vi "Data Logging Application.vi"() -> ()   [LabVIEW 2014]
doc: "This application allows the user to save any variables on the shared variable engine (NI SVE) in a TDMS file."
uses:
  <vilib>/Utility/miscctls.llb/LVRectTypeDef.ctl
  TypeDef/Q1 Message.ctl
  Support/Data Logger Global Variable.vi
  Supporting Folder/DV Prototype Global Variables.vi
  Support/Data logger Array Enqueue Function.vi
  Support/Global Variables/Recording Stop Watch.vi
  Support/Data logger Scalar Enqueue Function.vi
  <vilib>/Utility/NIReport.llb/NI_report.lvclass
  <userlib>/Notify Icon/Public/NotifyIcon.lvclass
panel:
  in  "DB Type":u16
  in  "delimiter":string=";"
  in  "Invisible Libraries":string[](array[string])
  in  "TDMS Properties":bool
  in  "Folder Setting":bool
  in  "Preference":bool
  in  "Description":string
  in  "Author":string
  in  "Title":string
  in  "Select All":bool
  in  "Auto Defrag":bool
  out "Date Time":string
  out "Application State":T1(ring)
  in  "Buffer size":u32=1000 min=1 step=1 format="%d data"
  in  "create database":bool
  out "Database Status":string
  in  "Deployed Libraries":i32[](listbox)
  in  "Server Name":string="localhost"
  in  "Add date/time to file name":bool
  in  "File Name":string="data log 1"
  out "Registered file name":string="data log 1" caption="Registered File Name"
  in  "database folder":path=path "C:/Ehsan Temp Folder/TFS/LV/Data Logging with LabVIEW/Database"
  in  "Folder to store TDMS file":path=path "C:/Ehsan Temp Folder/TFS/LV/Data Logging with LabVIEW/TDMS files"
  in  "View":bool
  in  "Initialize":bool
  in  "Stop Button":bool
  in  "Record Button":bool
  out "Recording Time":dbl format="%.1f sec"
  in  "Sampling Period":u32=100 min=1 step=1 format="%.0f msec"
  in  "Exit Button":bool
  in  "Variables":i32[](listbox)
  # "Data Logging Application"
  # "Status"
  # "Setting"
  # "Controls"
  # "Variables"
  # "Data Logging Application © 2015 Ehsan Peymani. All rights reserved."
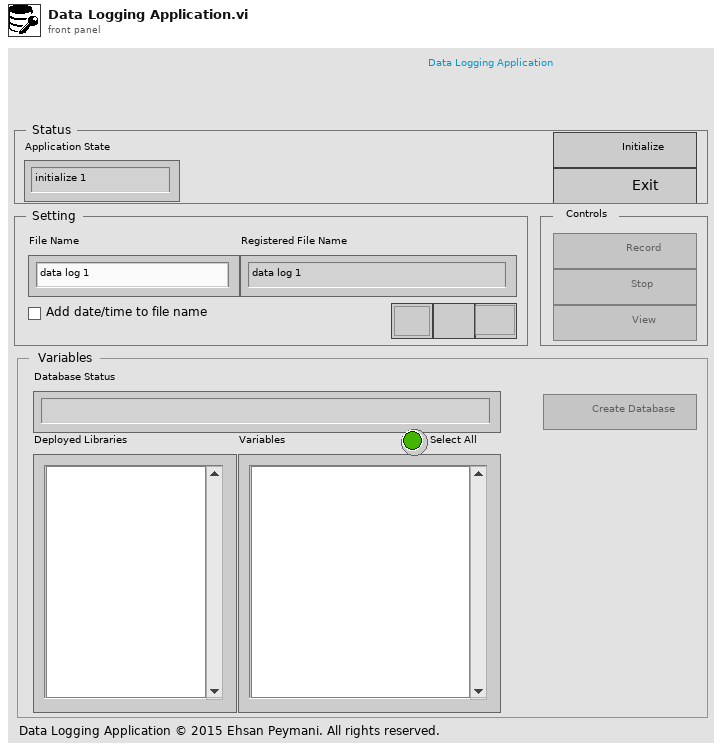
[diagram p1: front panel]
types:
  T1 = enum16{"initialize 1", "initialize 2", "initialize 3", "initialize 4", "initialize 5", "initialize 6", "initialize 7", "initialize 8", "initialize 9", "Idle", "Preparation 1", "Preparation 2", "Preparation 3", "Preparation 4", "Record", "Stop recording", "Exit", "Defrag", "View", "Create Database", "Update folder setting", "Update Preference", "Update TDMS properties", "CSV Delimiter", "DB Type", "Hidden Processes", "Replace Database", "Logged File Viewer", "Defrag Prompt File", "View Prompt File", "Save to config file", "Open from config file"}
  T2 = typedef "LVRectTypeDef.ctl" = cluster{"Left":i16, "Top":i16, "Right":i16, "Bottom":i16}
  T3 = enum16{"Config File", "Image File", "Word Template", "Release Note", "Help HTML", "Help Word", "Error List", "Excel Template", "CSV Template", "Tray Icon"}
  T4 = cluster{"Folder Path containing version information":path, "File name (including .ini)":path, "Section":string}
  T5 = typedef "LVPointTypeDef.ctl" = cluster{"Horizontal":i16, "Vertical":i16}
  T6 = cluster{"no. Displays":i32, "Display info - Menu":string[]}
  T7 = cluster{"path":path, "This VI":refnum<vi>, "Level of Application":u8}
  T8 = cluster{"Selected Variable Names":string[], "Selected Variable URL":string[], "Selected Variable Type":string[], "Container Variable Name":string[], "Container Variable URL":string[], "Selected Library URL":string[], "Library Name":string[], "Library URL":string[], "TDMS ref":refnum<k34>, "TDMS file path":path, "DB path array":path[], "DB availability for selected":bool[], "Selected Variables":i32[], "Bool Control Ref":refnum<vi>[], "Seetings ref":refnum<vi>[]}
  T9 = cluster{"String":refnum<vi>[], "Numeric":refnum<vi>[], "Path":refnum<vi>[], "Boolean":refnum<vi>[]}
  T10 = cluster{"Q2_scalar":refnum<queue>, "Q2_1Darray":refnum<queue>, "Q2_2Darray":refnum<queue>}
  T11 = enum32{"Invalid", "Standard", "Closed", "Hidden", "Minimized", "Maximized"}
  T12 = enum16{"Config File", "Image File", "Word Template", "Release Note", "Help HTML", "Help Word", "Error List", "Excel Template", "CSV Template"}
  T13 = typedef "Q1 Message.ctl" = cluster{"state":enum16{"initialize 1", "initialize 2", "initialize 3", "initialize 4", "initialize 5", "initialize 6", "initialize 7", "initialize 8", "initialize 9", "Idle", "Preparation 1", "Preparation 2", "Preparation 3", "Preparation 4", "Record", "Stop recording", "Exit", "Defrag", "View", "Create Database", "Update folder setting", "Update Preference", "Update TDMS properties", "CSV Delimiter", "DB Type", "Hidden Processes", "Replace Database", "Logged File Viewer", "Defrag Prompt File", "View Prompt File", "Save to config file", "Open from config file"}, "data":variant}
  T14 = enum16{"Standard Report", "HTML", "Word", "Excel"}
  T15 = enum16{"maximized", "minimized", "normal", "no change"}
  T16 = enum16{"Config File", "Image File", "Word Template", "Release Note", "Help HTML", "Help Word", "Error List", "Excel Template", "CSV Template", "Tray Icon", "Data Viewer"}
  T17 = typedef "sizeaction.ctl" = enum32{"Minimized", "Maximized", "Resized"}
  T18 = cluster{"Title":string, "Title":string, "Icon":i32, "Timeout (ms)":i32}
  T19 = typedef "Notify Icon.lvclass/Notify Event Type.ctl" = enum16{"<Invalid Event>", "Tray Icon Click", "Tray Icon DoubleClick", "BalloonTip Shown", "BalloonTip Clicked", "BalloonTip Closed", "Menu Item Clicked"}
  T20 = typedef "eventvkey.ctl" = enum16{"ASCII", "Enter", "Return", "Shift", "Ctrl", "Alt", "Cmd", "Opt", "Caps", "NumLock", "Clear", "Break", "Up", "Down", "Left", "Right", "Insert", "Delete", "Home", "End", "PageUp", "PageDown", "Escape", "Help", "Pause", "ScrollLock", "F1", "F2", "F3", "F4", "F5", "F6", "F7", "F8", "F9", "F10", "F11", "F12", "F13", "F14", "F15", "F16", "F17", "F18", "F19", "F20", "F21", "F22", "F23", "F24", "Play", "VolumeUp", "VolumeDown", "Mute", "Two Byte Char"}
  T21 = cluster{"Shift":bool, "Ctrl":bool, "Alt":bool, "Cmd":bool, "Opt":bool}
  T22 = enum8{"Enabled", "Disabled", "Disabled and Grayed Out"}
  T23 = enum16{"open", "open or create", "create or replace", "create", "open (read-only)"}
  T24 = cluster{"Library Name":string[], "library URL":string[]}
  T25 = cluster{"Variable Name":string[], "Variable URL":string[], "Variable Type":string[], "Variable Type Code":i32[]}
  T26 = cluster{"Sampling Period":u32, "TDMS ref":refnum<k34>, "Selected Variable URL":string[], "Selected Variable Type":string[], "Selected Variable Names":string[]}
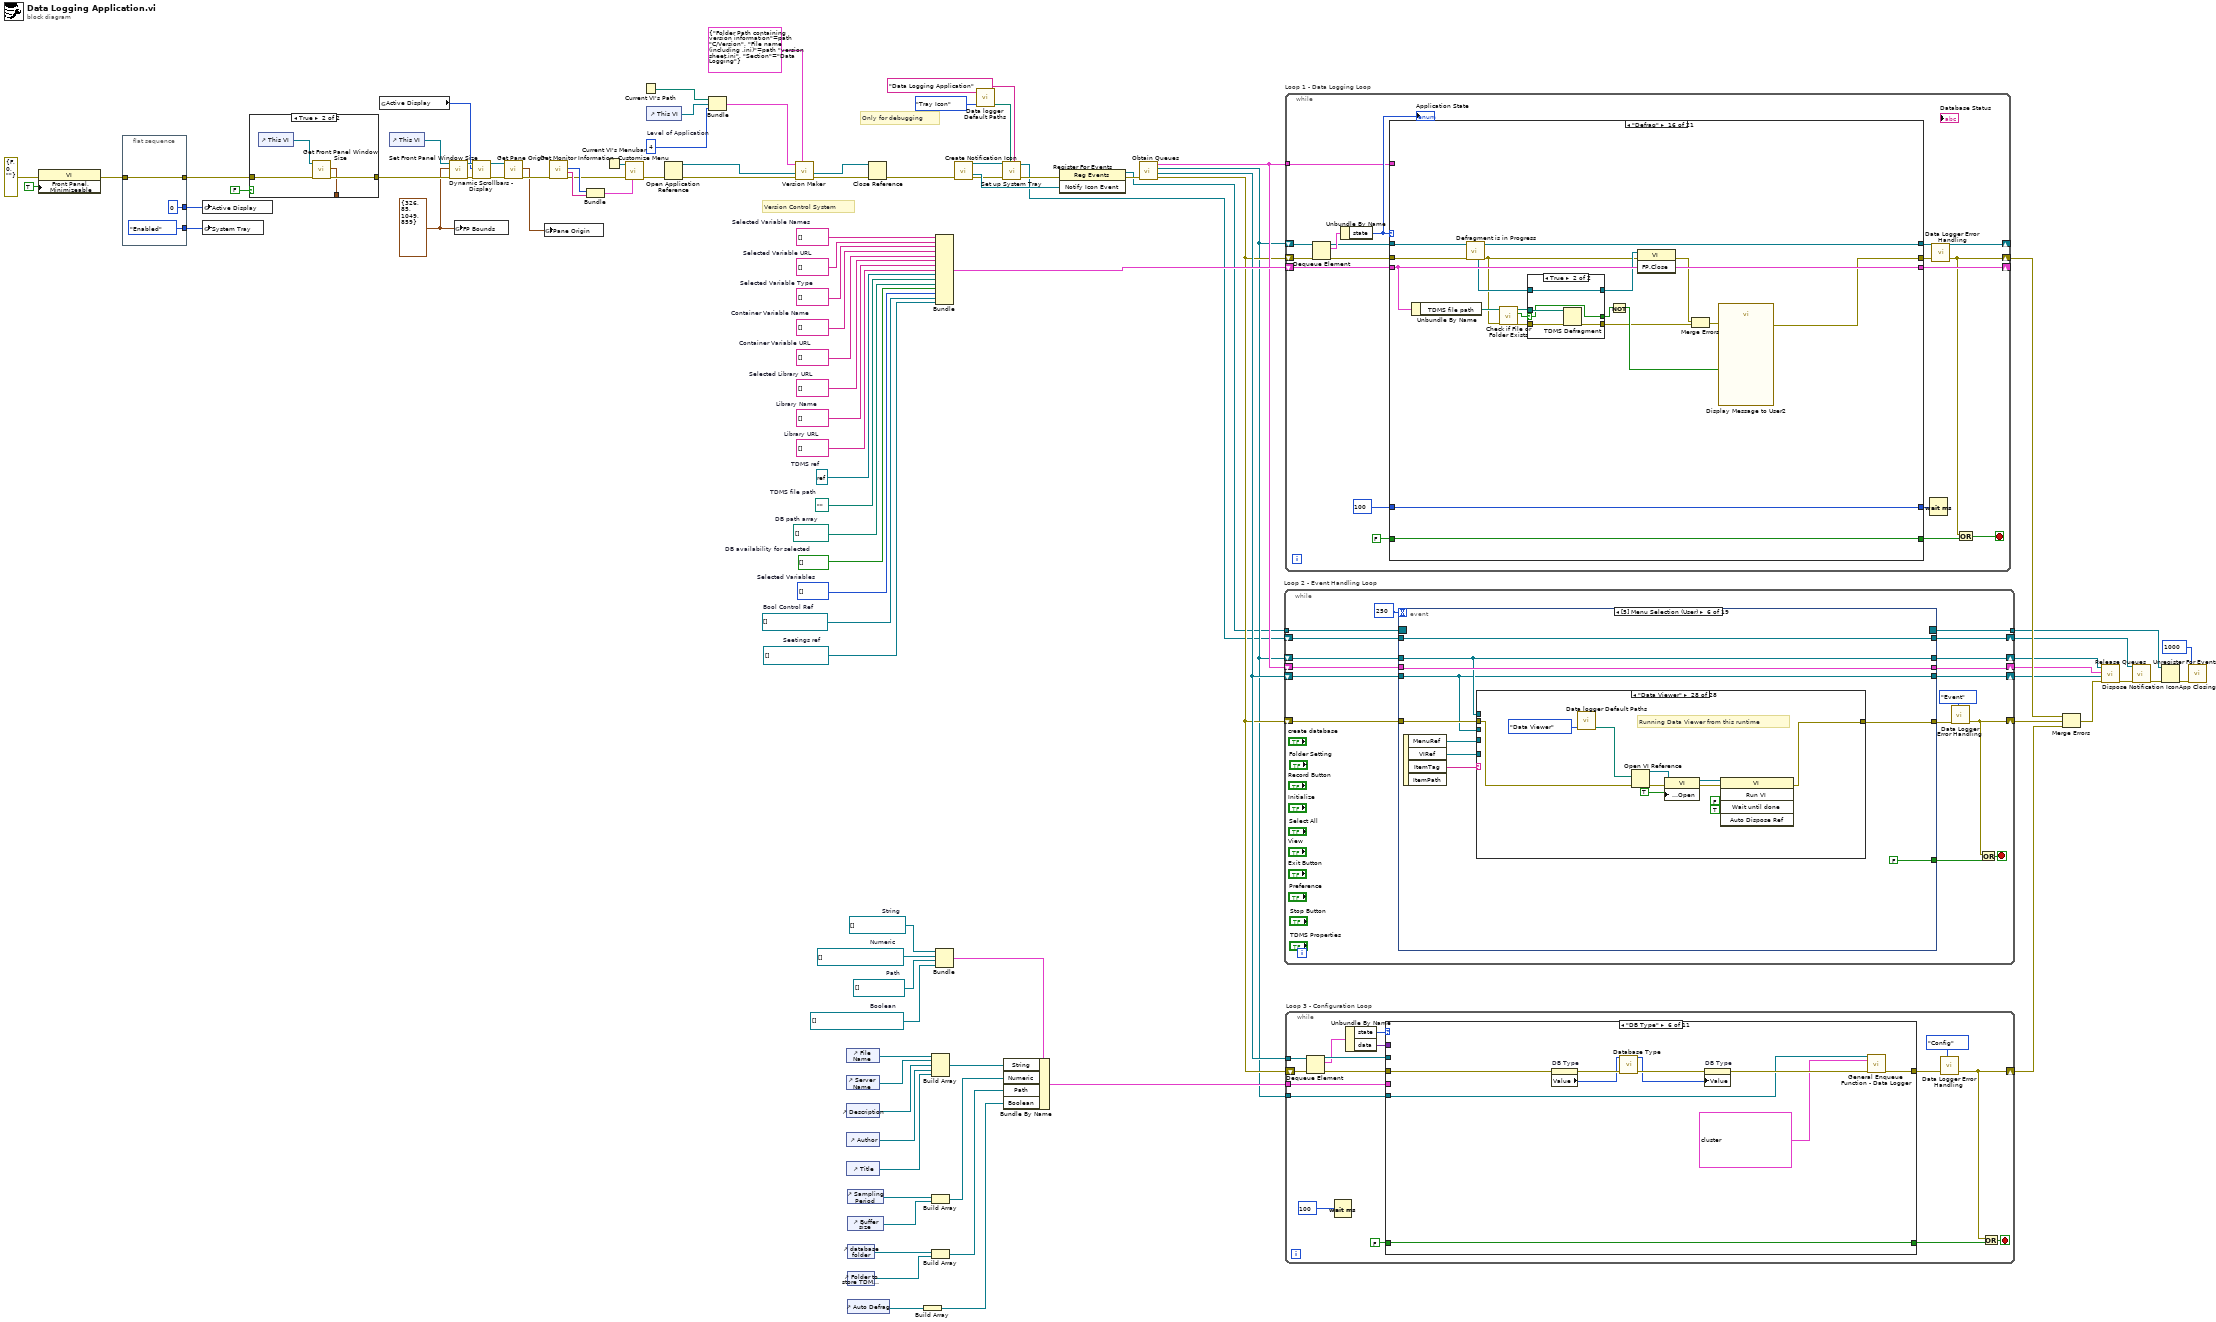
[diagram p0: block diagram]
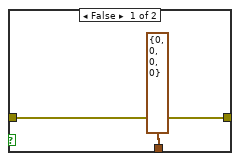
[diagram p2: hidden frame]
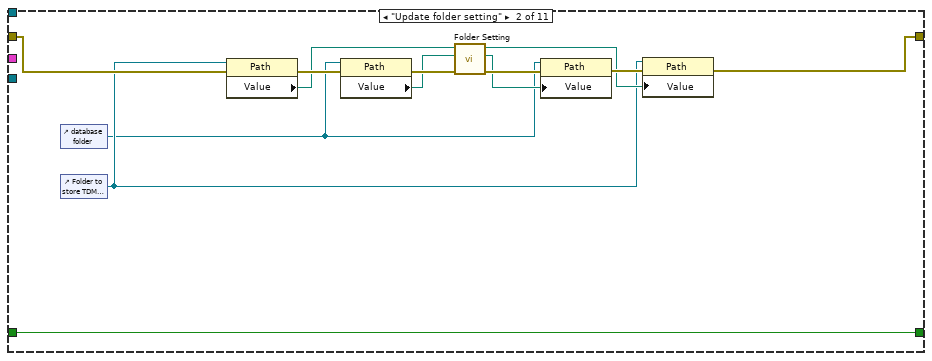
[diagram p4: hidden frame]
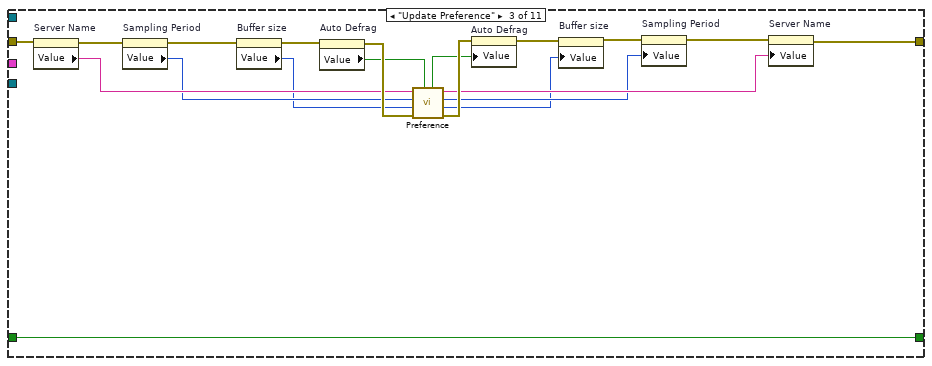
[diagram p5: hidden frame]
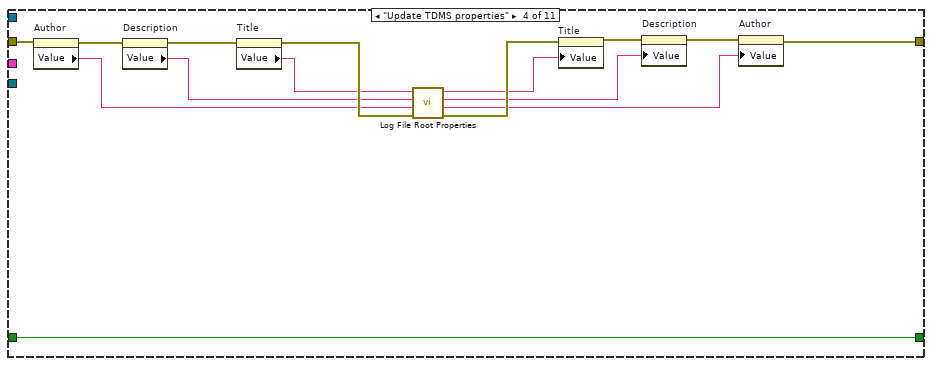
[diagram p6: hidden frame]
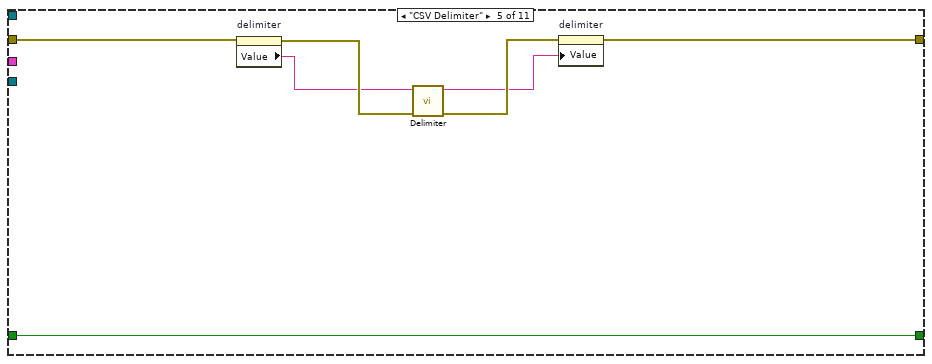
[diagram p7: hidden frame]
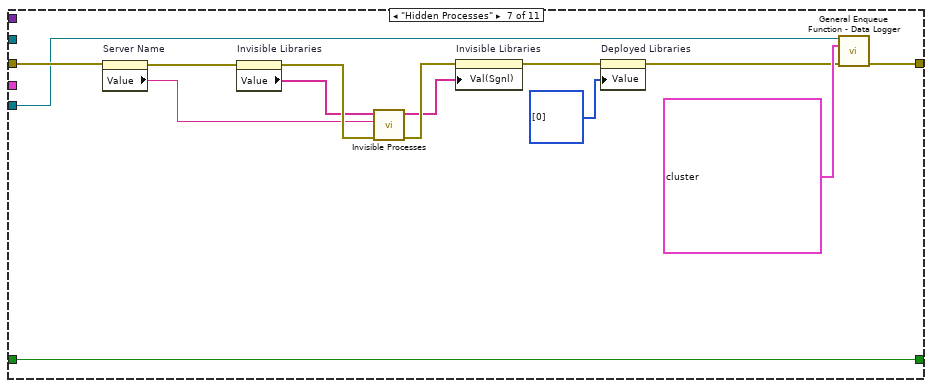
[diagram p8: hidden frame]
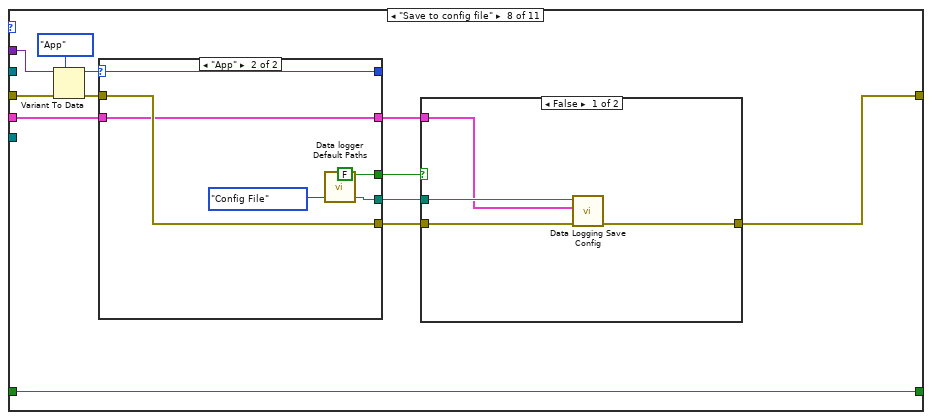
[diagram p9: hidden frame]
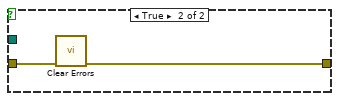
[diagram p10: hidden frame]
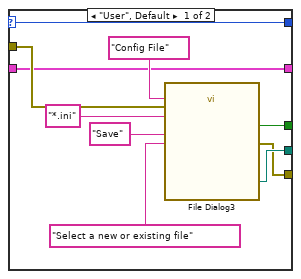
[diagram p11: hidden frame]
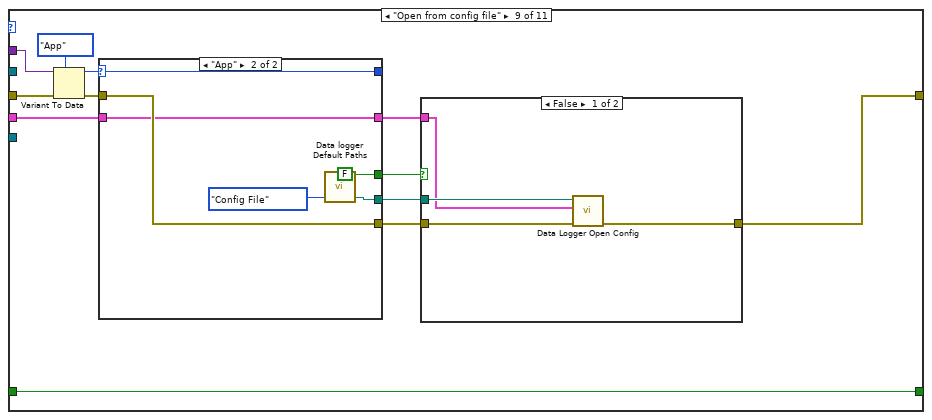
[diagram p12: hidden frame]
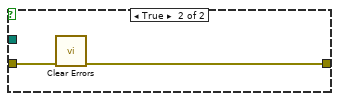
[diagram p13: hidden frame]
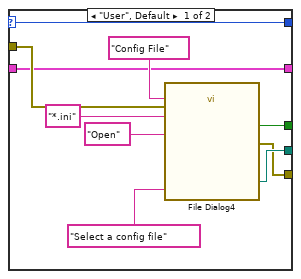
[diagram p14: hidden frame]
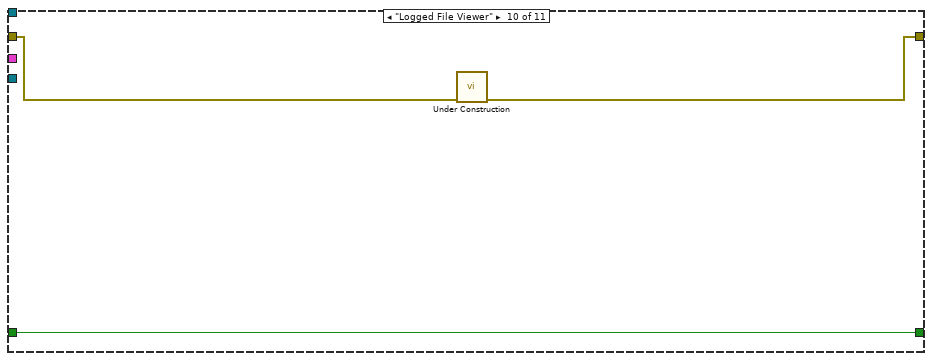
[diagram p15: hidden frame]
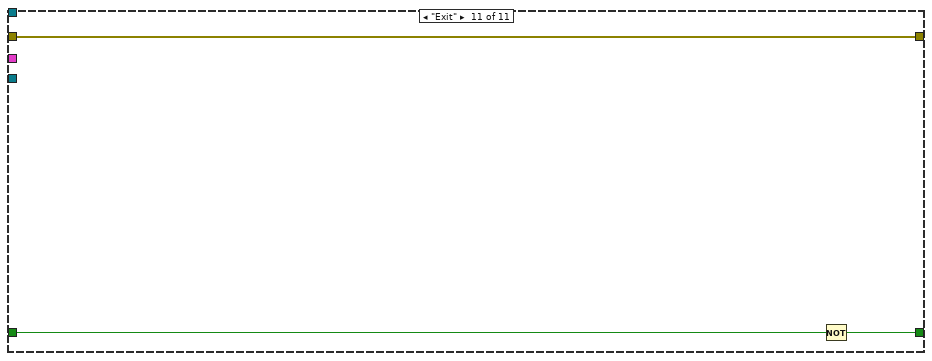
[diagram p16: hidden frame]
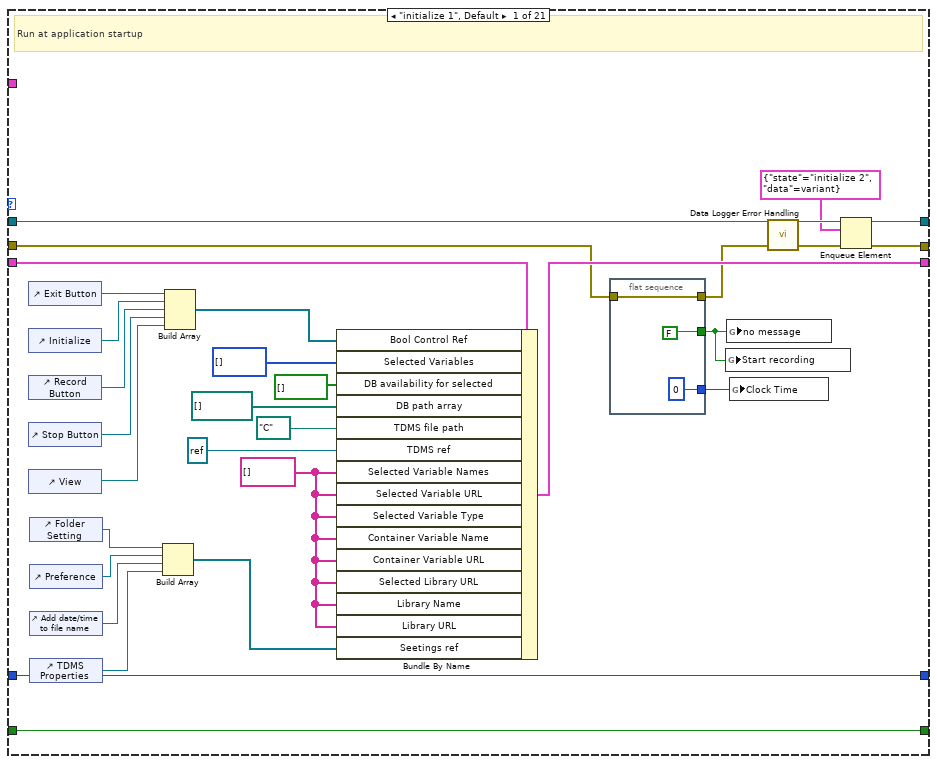
[diagram p17: hidden frame]
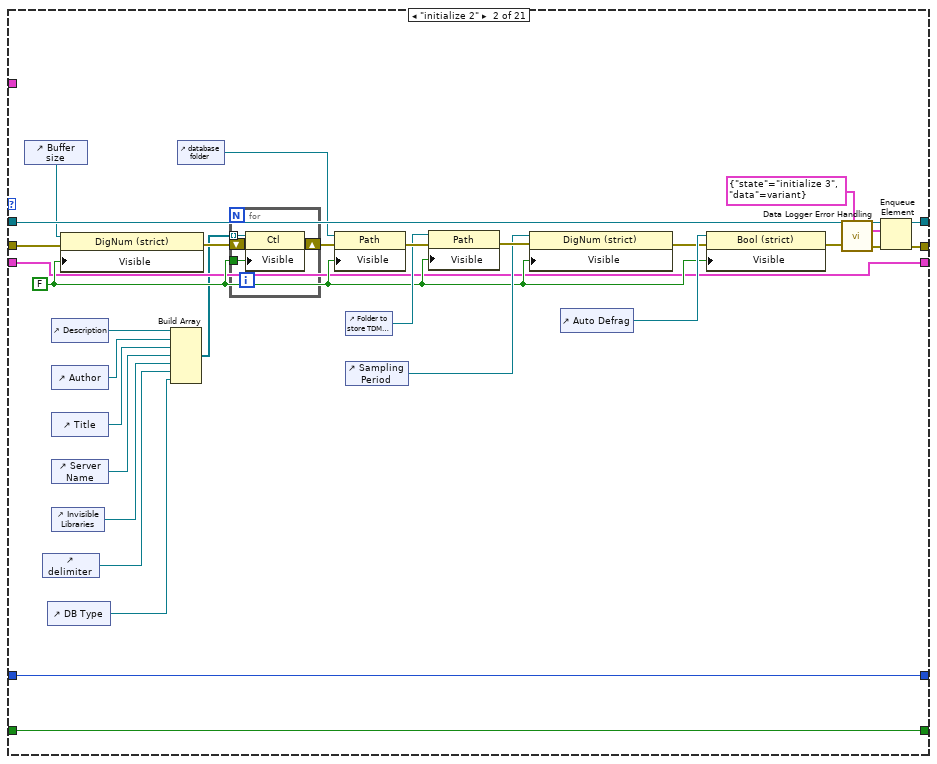
[diagram p18: hidden frame]
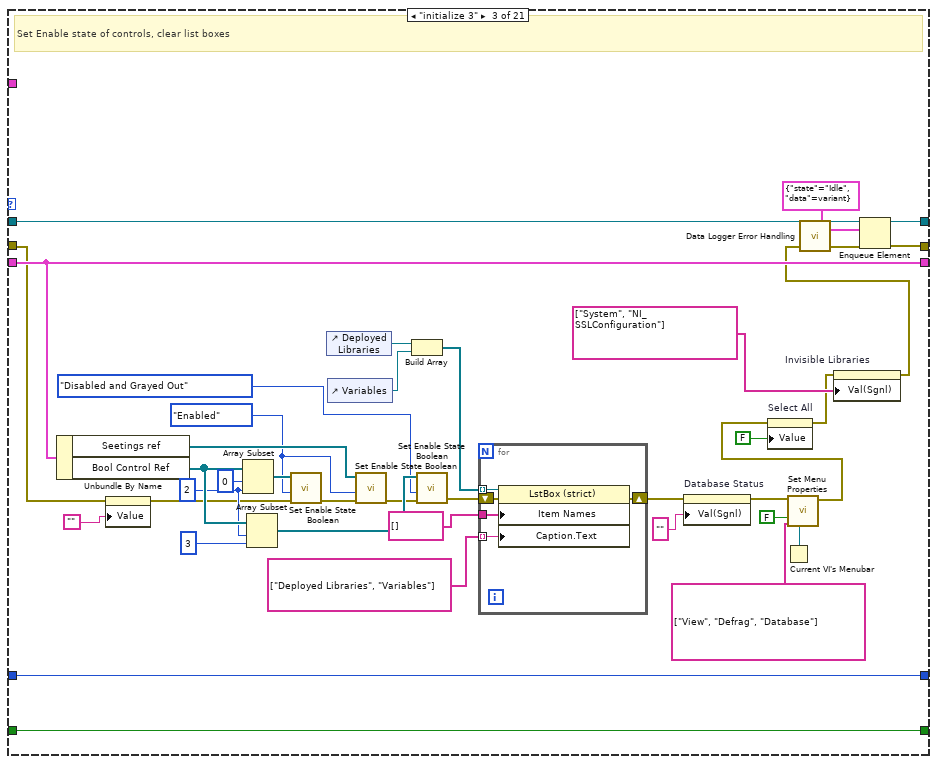
[diagram p19: hidden frame]
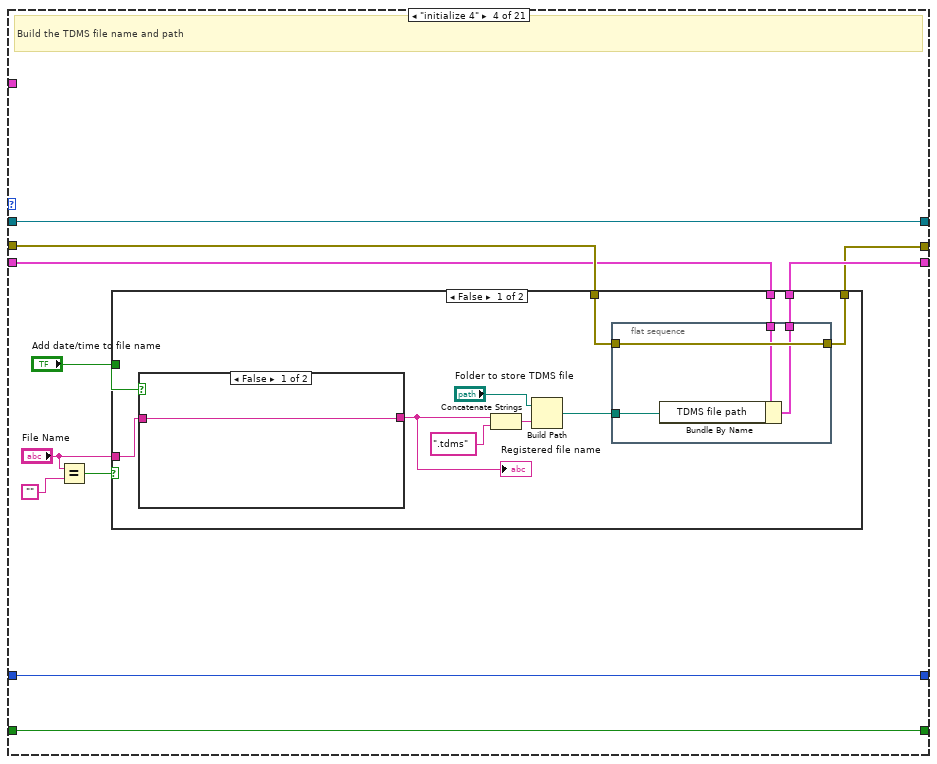
[diagram p20: hidden frame]
diagram:
  w5 = refnum<vi>[] []  # Seetings ref
  w7 = T2 {"Left"=326, "Top"=85, "Right"=1049, "Bottom"=859} ("Front Panel Window:Window Bounds")
  w45 = refnum<vi>[] []  # Boolean
  w48 = refnum<vi>[] []  # Numeric
  w51 = refnum<vi>[] []  # Path
  w54 = refnum<vi>[] []  # String
  w71 = string[] []  # Container Variable URL
  w80 = refnum<vi>[] []  # Bool Control Ref
  w75 = refnum<k34> refnum  # TDMS ref
  w79 = i32[] []  # Selected Variables
  w78 = bool[] []  # DB availability for selected
  w77 = path[] []  # DB path array
  w76 = path ""  # TDMS file path
  w74 = string[] []  # Library URL
  w73 = string[] []  # Library Name
  w72 = string[] []  # Selected Library URL
  w82 = string[] []  # Container Variable Name
  w83 = string[] []  # Selected Variable Type
  w84 = string[] []  # Selected Variable URL
  w85 = string[] []  # Selected Variable Names
  w88 = u8 4  # Level of Application
  # "Only for debugging"
  # "Version Control System"
  n1 = property class="VI"(error in=errorcluster {"status"=FALSE, "code"=0, "source"=""} ("error constant"), "Front Panel.Minimizeable"=TRUE ("Front Panel Window:Minimizable")) -> (error out=w4:errorcluster)  [unwired: 1 in, 1 out]
  n2 = flat-sequence {
    tunnel: [u16 0 ("Active Display")] -> w23
    tunnel: [enum16{"Enabled", "Disabled"}."Enabled" ("System Tray")] -> w22
    tunnel: [w97] -> w10
    tunnel: w4 -> [w97]
    frame #0 {
    }
  }
  n3 = global write "Data Logger Global Variable.vi" "Active Display"(w23) -> ()
  n4 = global write "Data Logger Global Variable.vi" "System Tray"(w22) -> ()
  n5 = case shown="True" FALSE {
    tunnel: w10 -> [w101 w104]
    tunnel: [w101 w103] -> w12
    tunnel: [T2 {"Left"=0, "Top"=0, "Right"=0, "Bottom"=0} ("Front Panel Window:Window Bounds") w102] -> _
    frame False {
    }
    frame True {
      n6 = control-ref of="This VI"() -> (w105:refnum<vi>)
      n7 = call "Get Front Panel Window Size.vi"("error in"=w104, "VI Ref"=w105) -> ("error out"=w103:errorcluster, "FP:Window Bounds"=w102:T2)  [unwired: 4 in, 4 out]
    }
  }
  n8 = global read "DV Prototype Global Variables.vi" "Active Display"() -> (w13:u16)
  n9 = control-ref of="This VI"() -> (w19:refnum<vi>)
  n10 = call "Set Front Panel Window Size.vi"("error in"=w12, "Front Panel Window:Window Bounds"=w7, "VI Ref"=w19) -> ("error out"=w21:errorcluster, "VI Ref"=w20:refnum<vi>)  [unwired: 7 in]
  n11 = global write "Data Logger Global Variable.vi" "FP Bounds"(w7) -> ()
  n12 = call "Dynamic Scrollbars - Display.vi"("error in"=w21, "Active Display in"=w13, "VI Ref"=w20) -> ("error out"=w18:errorcluster, "VI Ref"=w17:refnum<vi>)  [unwired: 6 in, 1 out]
  n13 = call "Get Pane Origin.vi"("error in"=w18, "VI Ref"=w17) -> ("error out"=w16:errorcluster, "Pane Origin"=w6:T5[])  [unwired: 7 in, 1 out]
  n14 = global write "Data Logger Global Variable.vi" "Pane Origin"(w6) -> ()
  n15 = call "Get Monitor Information.vi"("error in"=w16) -> ("error out"=w11:errorcluster, "Display info - Menu"=w14:string[], "no. Displays"=w15:i32)  [unwired: 6 in, 2 out]
  n16 = Bundle("no. Displays"=w15, "Display info - Menu"=w14) -> (w8:T6)  [unwired: 1 in]
  n17 = Current VI's Menubar() -> (w70:refnum<k9>)
  n18 = call "Customize Menu.vi"("Display information"=w8, "error in"=w11, "menu reference"=w70) -> ("error out"=w69:errorcluster)  [unwired: 8 in]
  n19 = Current VI's Path() -> (path=w86:path)
  n20 = control-ref of="This VI"() -> (w87:refnum<vi>)
  n21 = Open Application Reference(8:w69) -> (0:w94:errorcluster, 3:w91:refnum<vi>)  [unwired: 3 in]
  n22 = Bundle("path"=w86, "This VI"=w87, "Level of Application"=w88) -> (w89:T7)  [unwired: 1 in]
  n23 = call "Version Maker.vi"("Version Sheet Cluster"=T4 {"Folder Path containing version information"=path "C:/Version", "File name (including .ini)"=path "version sheet.ini", "Section"="Data Logging"}, "Error In"=w94, "Open Application Reference in"=w91, "VI Information"=w89) -> ("Error Out"=w93:errorcluster, "Open Application Reference out"=w90:refnum<vi>)  [unwired: 4 in, 2 out]
  n24 = control-ref of="File Name"() -> (w60:refnum<vi>)
  n25 = control-ref of="Server Name"() -> (w59:refnum<vi>)
  n26 = control-ref of="Description"() -> (w43:refnum<vi>)
  n27 = control-ref of="Author"() -> (w42:refnum<vi>)
  n28 = control-ref of="Title"() -> (w41:refnum<vi>)
  n29 = control-ref of="Sampling Period"() -> (w58:refnum<vi>)
  n30 = control-ref of="Buffer size"() -> (w57:refnum<vi>)
  n31 = control-ref of="database folder"() -> (w56:refnum<vi>)
  n32 = control-ref of="Folder to store TDMS file"() -> (w55:refnum<vi>)
  n33 = control-ref of="Auto Defrag"() -> (w46:refnum<vi>)
  n34 = Close Reference(reference=w90, error in (no error)=w93) -> (error out=w33:errorcluster)
  n35 = Build Array(w46) -> (w44:refnum<vi>[])
  n36 = Build Array(w60, w59, w43, w42, w41) -> (w53:refnum<vi>[])
  n37 = Build Array(w58, w57) -> (w47:refnum<vi>[])
  n38 = Build Array(w56, w55) -> (w50:refnum<vi>[])
  n39 = Bundle("Selected Variable Names"=w85, "Selected Variable URL"=w84, "Selected Variable Type"=w83, "Container Variable Name"=w82, "Container Variable URL"=w71, "Selected Library URL"=w72, "Library Name"=w73, "Library URL"=w74, "TDMS ref"=w75, "TDMS file path"=w76, "DB path array"=w77, "DB availability for selected"=w78, "Selected Variables"=w79, "Bool Control Ref"=w80, "Seetings ref"=w5) -> (w81:T8)  [unwired: 1 in]
  n40 = Bundle("String"=w54, "Numeric"=w48, "Path"=w51, "Boolean"=w45) -> (w52:T9)  [unwired: 1 in]
  n41 = call <userlib>:"Create Notification Icon.vi"("error in (no error)"=w33) -> ("NotifyIcon out"=w37:refnum<class "NotifyIcon.lvclass">, "Notify Icon Event"=w39:refnum<user-event>, "error out"=w38:errorcluster)  [unwired: 12 out]
  n42 = call "Data logger Default Paths.vi"("Path Type"=T3."Tray Icon") -> ("Path"=w31:path)  [unwired: 4 in]
  n43 = call "Set up System Tray.vi"("Icon Tip Strip Text"="Data Logging Application", "Image Path"=w31, "error in"=w38, "NotifyIcon in"=w37) -> ("error out"=w35:errorcluster, "NotifyIcon out"=w29:refnum<class "NotifyIcon.lvclass">)  [unwired: 6 in]
  n44 = Bundle By Name(cluster=w52, "String"=w53, "Numeric"=w47, "Path"=w50, "Boolean"=w44) -> (w49:T9)
  n45 = register-events(error in=w35, w39) -> (reference out=w30:refnum<event-registration>, error out=w34:errorcluster)  [unwired: 1 in]
  n46 = call "Obtain Queues.vi"("error in (no error)"=w34) -> ("error out"=w62:errorcluster, "Q3"=w63:refnum<queue>, "Q1"=w40:refnum<queue>, "Q2 Cluster"=w68:T10)  [unwired: 7 in]
  n47 = while "Loop 2 - Event Handling Loop" {
    shift-right: [w120] -> w66
    shift-left: w40 -> [w122]
    shift-right: [w111] -> w95
    shift-left: w62 -> [w121]
    shift-right: [w118] -> w65
    shift-left: w68 -> [w119]
    shift-right: [w113] -> w64
    shift-left: w63 -> [w114]
    tunnel: w30 -> [w109]
    shift-right: [w107] -> w25
    shift-left: w29 -> [w108]
    tunnel: [w106] -> w24
    stop <- w116 stop-if-true
    n48 = event shown="[5] Menu Selection (User)" {
      selector: w109 -> [_ _ _ _ _ _ _ _ _ _ _ _ _ _ _ _ _ _ _]
      dyn-events: [_ _ _ _ _ _ _ _ _ _ _ _ _ _ _ _ _ _ _] -> w106
      timeout: u32 250 ("milliseconds to wait") -> [_ _ _ _ _ _ _ _ _ _ _ _ _ _ _ _ _ _ _]
      tunnel: w122 -> [w134 w154 w163 w199 w242 w360 w563 w585 w595 w604 w613 w625 w637 w642 w654 w662 w670 w678 w701]
      tunnel: w121 -> [w128 w149 w160 w196 w244 w362 w576 w580 w590 w602 w612 w621 w636 w646 w650 w658 w666 w674 w690]
      tunnel: [_ _ _ _ w238 FALSE TRUE FALSE FALSE FALSE _ _ _ _ _ _ _ _ _] -> w117
      tunnel: [w134 w154 w163 w199 w242 w360 w562 w586 w595 w605 w616 w627 w638 w642 w654 w662 w670 w678 w701] -> w120
      tunnel: [w131 w149 w159 w195 w243 w361 w565 w584 w594 w607 w614 w628 w635 w643 w653 w661 w669 w673 w698] -> w112
      tunnel: w119 -> [w133 w153 w162 w198 w241 w364 w577 w587 w593 w608 w617 w631 w639 w647 w655 w663 w671 w677 w700]
      tunnel: [w133 w153 w162 w198 w241 w364 w577 w587 w593 w608 w617 w631 w639 w647 w655 w663 w671 w677 w700] -> w118
      tunnel: w114 -> [w124 w152 w161 w197 w240 w359 w575 w581 w591 w598 w611 w622 w633 w641 w652 w660 w668 w676 w699]
      tunnel: [w124 w152 w161 w197 w240 w359 w567 w581 w591 w598 w611 w622 w633 w641 w651 w659 w667 w676 w699] -> w113
      tunnel: w108 -> [w123 w151 w158 w194 w236 w357 w561 w579 w589 w597 w610 w618 w632 w640 w648 w656 w664 w672 w689]
      tunnel: [w123 w151 w157 w193 w236 w357 w561 w579 w589 w597 w610 w618 w632 w640 w648 w656 w664 w672 w689] -> w107
      event Timeout {
        n49 = event-data() -> ()  [unwired: 1 in, 2 out]
        n50 = flat-sequence {
          tunnel: [w136] -> w125
          tunnel: w128 -> [w135]
          tunnel: [w135] -> w126
          frame #0 {
            n51 = Get Date/Time In Seconds() -> (seconds since 1Jan1904=w137:timestamp)
            n52 = Format Date/Time String(time format string (%c)="%Y-%m-%d  %H:%M:%S", seconds (now)=w137) -> (date/time string=w136:string)  [unwired: 1 in]
          }
        }
        n53 = global read "Recording Stop Watch.vi" "Start recording"() -> (w132:bool)
        n54 = case shown="False" w132 {
          tunnel: [0.0 w144] -> w129
          tunnel: [FALSE TRUE] -> w130
          tunnel: [w139 w142] -> w127
          tunnel: w126 -> [w139 w142]
          frame False {
          }
          frame True {
            n55 = global read "Recording Stop Watch.vi" "Clock Time"() -> (w147:u32)
            n56 = Tick Count (ms)() -> (millisecond timer value=w148:u32)
            n57 = Subtract(x=w148, y=w147) -> (x-y=w146:u32)
            n58 = Divide(x=w146, y=u32 1000) -> (x/y=w144:dbl)
          }
        }
        "Recording Time" <- w129
        n59 = property on="Recording Time" class="DigNum (strict)"(error in=w127, "Visible"=w130) -> (error out=w131:errorcluster)  [unwired: 1 in, 1 out]
        "Date Time" <- w125
      }
      event Panel Close? {
        n60 = event-data() -> ()  [unwired: 1 in, 4 out]
        n61 = event-data("Discard?"=TRUE) -> ()  [unwired: 1 in, 1 out]
      }
      event Panel Resize {
        n62 = event-data() -> ("VIRef"=w156:refnum<vi>, "Act"=w155:T17)  [unwired: 1 in]
        n63 = case shown="\"Minimized\", Default" w155 {
          tunnel: w156 -> [w164 w183 w189]
          tunnel: w158 -> [w175 w180 w190]
          tunnel: w160 -> [w167 w182 w186]
          tunnel: [w176 w181 w191] -> w159
          tunnel: [w169 w180 w190] -> w157
          frame "Minimized", Default {
            w172 = 1 items=["None", "Info", "Warning", "Error"] ("Icon")
            n64 = property class="VI"(reference=w164, error in=w167, "Front Panel.Minimizeable"=FALSE ("Front Panel Window:Minimizable")) -> (error out=w166:errorcluster)  [unwired: 1 out]
            n65 = global read "Data Logger Global Variable.vi" "System Tray"() -> (w168:enum16{"Enabled", "Disabled"})
            n66 = Bundle("Title"="Data Logging Application", "Title"="Data Logging Application is running. Click on this icon to bring it up. ", "Icon"=w172, "Timeout (ms)"=2500) -> (w170:T18)  [unwired: 1 in]
            n67 = call "Front Panel to System Tray.vi"("Balloon Tip Information"=w170, "Mode"=w168, "error in"=w166, "VIRef"=w164, "NotifyIcon"=w175) -> ("error out"=w176:errorcluster, "NotifyIcon"=w169:refnum<class "NotifyIcon.lvclass">)  [unwired: 5 in]
          }
          frame "Maximized" {
            n68 = global read "Data Logger Global Variable.vi" "Pane Origin"() -> (w177:T5[])
            n69 = global read "Data Logger Global Variable.vi" "FP Bounds"() -> (w178:T2)
            n70 = global read "Data Logger Global Variable.vi" "Active Display"() -> (w179:u16)
            n71 = call "Reset Front Panel.vi"("Active Display"=w179, "error in"=w182, "Pane Origin"=w177, "Front Panel Bounds"=w178, "VI Ref"=w183) -> ("error out"=w181:errorcluster)  [unwired: 5 in, 1 out]
          }
          frame "Resized" {
            n72 = global read "Data Logger Global Variable.vi" "FP Bounds"() -> (w184:T2)
            n73 = call "Get Front Panel Window Size.vi"("error in"=w186, "VI Ref"=w189) -> ("error out"=w187:errorcluster, "FP:Window Bounds"=w185:T2, "VI Ref"=w188:refnum<vi>)  [unwired: 4 in, 3 out]
            n74 = call "Dynamic Scrollbars - Resize Front Panel.vi"("error in"=w187, "OrgBnds"=w184, "NewBnds"=w185, "VI Ref"=w188) -> ("error out"=w191:errorcluster)  [unwired: 6 in, 1 out]
          }
        }
      }
      event User Event {
        n75 = event-data() -> ("Type"=w192:T19)  [unwired: 1 in]
        n76 = case shown="\"Tray Icon Click\"" w192 {
          tunnel: w196 -> [w201 w205 w227 w229 w231 w233 w235]
          tunnel: [w201 w210 w227 w229 w231 w233 w235] -> w195
          tunnel: [w200 w209 w226 w228 w230 w232 w234] -> w193
          tunnel: w194 -> [w200 w208 w226 w228 w230 w232 w234]
          frame "<Invalid Event>", Default {
          }
          frame "Tray Icon Click" {
            n77 = control-ref of="This VI"() -> (w203:refnum<vi>)
            n78 = property class="VI"(reference=w203, error in=w205, "Front Panel.Minimizeable"=TRUE ("Front Panel Window:Minimizable")) -> (reference out=w202:refnum<vi>, error out=w206:errorcluster)
            n79 = property class="VI"(reference=w202, error in=w206) -> (reference out=w216:refnum<vi>, error out=w215:errorcluster, "FP.State"=w217:T11)
            n80 = case shown="\"Hidden\"" w217 {
              tunnel: w216 -> [w219 w225]
              tunnel: w215 -> [w218 w224]
              tunnel: T11."Standard" ("State") -> [_ w222]
              tunnel: [w218 w221] -> w213
              tunnel: [w219 w220] -> w212
              frame "Invalid", Default {
              }
              frame "Hidden" {
                n81 = invoke class="VI" method="FP.Open"(reference=w225, error in=w224, "Activate"=TRUE, "State"=w222) -> (reference out=w220:refnum<vi>, error out=w221:errorcluster)  [unwired: 1 in, 3 out]
              }
            }
            n82 = Close Reference(reference=w212, error in (no error)=w213) -> (error out=w211:errorcluster)
            n83 = call <userlib>:"Set Tray Icon Visibility.vi"("NotifyIcon in"=w208, "Show Tray Icon"=FALSE, "error in (no error)"=w211) -> ("NotifyIcon out"=w209:refnum<class "NotifyIcon.lvclass">, "error out"=w210:errorcluster)  [unwired: 11 out]
          }
          frame "Tray Icon DoubleClick" {
          }
          frame "BalloonTip Shown" {
          }
          frame "BalloonTip Clicked" {
          }
          frame "BalloonTip Closed" {
          }
          frame "Menu Item Clicked" {
          }
        }
      }
      event Key Down? {
        n84 = event-data() -> ("Char"=w247:i16, "VKey"=w248:T20, "PlatMods"=w249:T21)  [unwired: 1 in, 7 out]
        n85 = case shown="\"F1\"" w248 {
          tunnel: w247 -> [w344 _ _]
          tunnel: [w345 "" ("type") "" ("type")] -> w245
          tunnel: [w342 w347 w351] -> w250
          tunnel: w244 -> [w342 w347 w352]
          tunnel: T12."Help HTML" ("Path Type 2") -> [_ _ w349]
          frame "ASCII", Default {
            n86 = To Unsigned Byte Integer(number=w344) -> (unsigned 8bit integer=w343:u8)
            n87 = Type Cast(type="a", x=w343) -> (*(type *) &x=w345:string)
          }
          frame "Enter" {
          }
          frame "F1" {
            n88 = call "Data logger Default Paths.vi"("Path Type"=w349) -> ("Path"=w353:path)  [unwired: 4 in]
            n89 = Control Online Help(1:w352, 2:w353, 4:enum16{"Contents", "Key", "Close"}."Contents" ("Operation")) -> (0:w351:errorcluster)  [unwired: 1 in]
          }
        }
        n90 = Unbundle By Name(w249) -> ("Ctrl"=w246:bool)
        n91 = case shown="True" w246 {
          tunnel: w245 -> [_ w260]
          tunnel: w250 -> [w252 w259]
          tunnel: [w252 w258] -> w243
          tunnel: w242 -> [_ w257]
          tunnel: w241 -> [_ w256]
          tunnel: w240 -> [_ w255]
          tunnel: FALSE -> [w251 w254]
          tunnel: [w251 w253] -> w238
          frame False {
          }
          frame True {
            n92 = case shown="\"E\", \"Q\", \"e\", \"q\"" w260 {
              tunnel: w259 -> [w262 w267 w273 w287 w298 w309 w322]
              tunnel: [w262 w263 w276 w290 w301 w312 w324] -> w258
              tunnel: w257 -> [_ _ w275 w289 w300 _ w323]
              tunnel: w256 -> [_ _ _ _ _ w311 _]
              tunnel: w255 -> [_ _ _ _ _ _ w325]
              tunnel: w254 -> [w261 w268 w274 w288 w299 w310 w319]
              tunnel: [w261 w268 w274 w288 w299 w310 w318] -> w253
              frame "False", Default {
              }
              frame "A", "a" {
                n93 = property on="Select All" class="Bool (strict)"(error in=w267) -> (error out=w264:errorcluster, "Value"=w266:bool)  [unwired: 1 in, 1 out]
                n94 = Not(x=w266) -> (.not. x?=w265:bool)
                n95 = property on="Select All" class="Bool (strict)"(error in=w264, "Val(Sgnl)"=w265) -> (error out=w263:errorcluster)  [unwired: 1 in, 1 out]
              }
              frame "I", "i" {
                n96 = control-ref of="Initialize"() -> (w272:refnum<vi>)
                n97 = property class="Bool"(reference=w272, error in=w273) -> (reference out=w269:refnum<vi>, error out=w270:errorcluster, "DisabledEnum"=w271:T22)
                n98 = case shown="\"Disabled\", Default" w271 {
                  tunnel: [w277 w283] -> w276
                  tunnel: w275 -> [_ w280]
                  tunnel: w270 -> [w277 w278]
                  tunnel: w269 -> [_ w279]
                  frame "Disabled", Default {
                  }
                  frame "Enabled" {
                    n99 = property class="Bool"(reference=w279, error in=w278, "Blinking"=FALSE) -> (error out=w282:errorcluster)  [unwired: 1 out]
                    n100 = call-poly "General Enqueue Function - Data Logger.vi"("QRef in"=w280, "Array of Messages"=T13[] [{"state"=enum."initialize 3", "data"=variant}, {"state"=enum."initialize 4", "data"=variant}, {"state"=enum."initialize 5", "data"=variant}, {"state"=enum."initialize 6", "data"=variant}, {"state"=enum."Idle", "data"=variant}], "Error in"=w282) -> ("Error out"=w283:errorcluster)  [unwired: 11 in, 1 out]
                  }
                }
              }
              frame "R", "r" {
                n101 = property on="Record Button" class="Bool"(error in=w287) -> (error out=w286:errorcluster, "DisabledEnum"=w285:T22)  [unwired: 1 in, 1 out]
                n102 = case shown="\"Enabled\"" w285 {
                  tunnel: [w291 w295] -> w290
                  tunnel: w289 -> [_ w294]
                  tunnel: w286 -> [w291 w292]
                  frame "Disabled", Default {
                  }
                  frame "Enabled" {
                    n103 = call-poly "General Enqueue Function - Data Logger.vi"("QRef in"=w294, "Array of Messages"=T13[] [{"state"=enum."Preparation 1", "data"=variant}, {"state"=enum."Preparation 2", "data"=variant}, {"state"=enum."Preparation 3", "data"=variant}, {"state"=enum."Preparation 4", "data"=variant}, {"state"=enum."Record", "data"=variant}], "Error in"=w292) -> ("Error out"=w295:errorcluster)  [unwired: 11 in, 1 out]
                  }
                }
              }
              frame "V", "v" {
                n104 = property on="View" class="Bool"(error in=w298) -> (error out=w297:errorcluster, "DisabledEnum"=w296:T22)  [unwired: 1 in, 1 out]
                n105 = case shown="\"Enabled\"" w296 {
                  tunnel: [w305 w306] -> w301
                  tunnel: w300 -> [w304 _]
                  tunnel: w297 -> [w303 w306]
                  frame "Enabled" {
                    n106 = call-poly "General Enqueue Function - Data Logger.vi"("QRef in"=w304, "Q1 Message"=T13 {"state"=enum."View", "data"=variant}, "Error in"=w303) -> ("Error out"=w305:errorcluster)  [unwired: 11 in, 1 out]
                  }
                  frame "Disabled", Default {
                  }
                }
              }
              frame "S", "s" {
                n107 = property on="Stop Button" class="Bool"(error in=w309) -> (error out=w307:errorcluster, "DisabledEnum"=w308:T22)  [unwired: 1 in, 1 out]
                n108 = case shown="\"Enabled\"" w308 {
                  tunnel: [w316 w317] -> w312
                  tunnel: w307 -> [w315 w317]
                  tunnel: w311 -> [w314 _]
                  frame "Enabled" {
                    n109 = call "Enqueue Q2.vi"("Q1 Message"=T13 {"state"=enum."Stop recording", "data"=variant}, "error in (no error)"=w315, "Queue Ref"=w314) -> ("error out"=w316:errorcluster)  [unwired: 5 in, 3 out]
                  }
                  frame "Disabled", Default {
                  }
                }
              }
              frame "E", "Q", "e", "q" {
                n110 = property on="Exit Button" class="Bool"(error in=w322) -> (error out=w321:errorcluster, "DisabledEnum"=w320:T22)  [unwired: 1 in, 1 out]
                n111 = case shown="\"Enabled\"" w320 {
                  tunnel: w321 -> [w334 w341]
                  tunnel: w325 -> [w332 _]
                  tunnel: [w331 w341] -> w324
                  tunnel: w323 -> [w328 _]
                  tunnel: w319 -> [w327 w340]
                  tunnel: [w326 w340] -> w318
                  frame "Enabled" {
                    n112 = To Variant(anything=enum16{"App", "User"}."App") -> (Variant=w337:variant)
                    n113 = Bundle By Name(cluster=T13 {"state"=enum."Save to config file", "data"=variant} ("Q1 Message"), "data"=w337) -> (w338:T13)
                    n114 = Build Array(w338, T13 {"state"=enum."Exit", "data"=variant} ("Q1 Message")) -> (w333:T13[])
                    n115 = call-poly "General Enqueue Function - Data Logger.vi"("QRef in"=w332, "Array of Messages"=w333, "Error in"=w334) -> ("Error out"=w330:errorcluster)  [unwired: 11 in, 1 out]
                    n116 = Not(x=w327) -> (.not. x?=w326:bool)
                    n117 = call-poly "General Enqueue Function - Data Logger.vi"("QRef in"=w328, "Array of Messages"=T13[] [{"state"=enum."Exit", "data"=variant}], "Error in"=w330) -> ("Error out"=w331:errorcluster)  [unwired: 11 in, 1 out]
                  }
                  frame "Disabled", Default {
                  }
                }
              }
            }
          }
        }
        n118 = event-data() -> ()  [unwired: 2 in, 1 out]
      }
      event Menu Selection (User) {
        n119 = event-data() -> ("MenuRef"=w356:refnum<k9>, "VIRef"=w355:refnum<vi>, "ItemTag"=w363:string)  [unwired: 1 in, 1 out]
        n120 = case shown="\"Data Viewer\"" w363 {
          selector: w363 -> [_ _ _ _ _ _ _ _ _ _ _ _ _ _ _ _ _ _ _ _ _ _ w486 w494 w508 w522 w536 _]
          tunnel: w362 -> [w365 w369 w371 w373 w378 w384 w389 w394 w399 w404 w409 w414 w419 w424 w429 w434 w444 w454 w459 w462 w474 w480 w488 w496 w510 w524 w538 w553]
          tunnel: [w365 w368 w370 w375 w380 w385 w390 w395 w400 w405 w410 w415 w420 w425 w430 w435 w445 w455 w458 w463 w471 w481 w487 w495 w509 w523 w537 w552] -> w361
          tunnel: w360 -> [_ _ _ w374 w379 _ _ _ _ _ _ w411 _ w421 w426 w431 _ _ _ _ _ _ _ _ _ _ _ _]
          tunnel: w359 -> [_ _ _ _ _ w381 w386 w391 w396 w401 w406 _ w416 _ _ _ w442 w452 _ _ _ _ _ _ _ _ _ _]
          tunnel: w356 -> [_ _ _ _ _ _ _ _ _ _ _ _ _ _ _ _ _ _ _ _ _ _ w483 w497 w511 w525 w539 _]
          tunnel: w355 -> [_ _ _ _ _ _ _ _ _ _ _ _ _ _ _ _ _ _ _ _ _ _ _ w498 w512 w526 w540 _]
          frame "False", Default {
          }
          frame "Release Note" {
            n121 = call "Data logger Default Paths.vi"("Path Type"=T12."Release Note") -> ("Path"=w367:path)  [unwired: 4 in]
            n122 = call "open in notepad.vi"("error in (no error)"=w369, "Path"=w367) -> ("error out"=w368:errorcluster)  [unwired: 9 in]
          }
          frame "About Data Logging Application" {
            n123 = call "About Data Logger.vi"("Error In"=w371) -> ("Error Out"=w370:errorcluster)  [unwired: 10 in]
          }
          frame "View Current TDMS file" {
            n124 = call-poly "General Enqueue Function - Data Logger.vi"("QRef in"=w374, "Array of Messages"=T13[] [{"state"=enum."View", "data"=variant}, {"state"=enum."Idle", "data"=variant}], "Error in"=w373) -> ("Error out"=w375:errorcluster)  [unwired: 11 in, 1 out]
          }
          frame "Defrag Current TDMS file" {
            n125 = call-poly "General Enqueue Function - Data Logger.vi"("QRef in"=w379, "Array of Messages"=T13[] [{"state"=enum."Defrag", "data"=variant}, {"state"=enum."Idle", "data"=variant}], "Error in"=w378, "Mode"=enum16{"Back", "Front", "Replace"}."Replace") -> ("Error out"=w380:errorcluster)  [unwired: 10 in, 1 out]
          }
          frame "Folder Setting" {
            n126 = call-poly "General Enqueue Function - Data Logger.vi"("QRef in"=w381, "Array of Messages"=T13[] [{"state"=enum."Update folder setting", "data"=variant}, {"state"=enum."Idle", "data"=variant}], "Error in"=w384, "Mode"=enum16{"Back", "Front", "Replace"}."Replace") -> ("Error out"=w385:errorcluster)  [unwired: 10 in, 1 out]
          }
          frame "Preference" {
            n127 = call-poly "General Enqueue Function - Data Logger.vi"("QRef in"=w386, "Array of Messages"=T13[] [{"state"=enum."Update Preference", "data"=variant}, {"state"=enum."Idle", "data"=variant}], "Error in"=w389, "Mode"=enum16{"Back", "Front", "Replace"}."Replace") -> ("Error out"=w390:errorcluster)  [unwired: 10 in, 1 out]
          }
          frame "Log File Properties" {
            n128 = call-poly "General Enqueue Function - Data Logger.vi"("QRef in"=w391, "Array of Messages"=T13[] [{"state"=enum."Update TDMS properties", "data"=variant}, {"state"=enum."Idle", "data"=variant}], "Error in"=w394, "Mode"=enum16{"Back", "Front", "Replace"}."Replace") -> ("Error out"=w395:errorcluster)  [unwired: 10 in, 1 out]
          }
          frame "CSV Delimiter" {
            n129 = call-poly "General Enqueue Function - Data Logger.vi"("QRef in"=w396, "Array of Messages"=T13[] [{"state"=enum."CSV Delimiter", "data"=variant}, {"state"=enum."Idle", "data"=variant}], "Error in"=w399, "Mode"=enum16{"Back", "Front", "Replace"}."Replace") -> ("Error out"=w400:errorcluster)  [unwired: 10 in, 1 out]
          }
          frame "Database Type" {
            n130 = call-poly "General Enqueue Function - Data Logger.vi"("QRef in"=w401, "Array of Messages"=T13[] [{"state"=enum."DB Type", "data"=variant}, {"state"=enum."Idle", "data"=variant}], "Error in"=w404, "Mode"=enum16{"Back", "Front", "Replace"}."Replace") -> ("Error out"=w405:errorcluster)  [unwired: 10 in, 1 out]
          }
          frame "Hidden Processes" {
            n131 = call-poly "General Enqueue Function - Data Logger.vi"("QRef in"=w406, "Array of Messages"=T13[] [{"state"=enum."Hidden Processes", "data"=variant}, {"state"=enum."Idle", "data"=variant}], "Error in"=w409, "Mode"=enum16{"Back", "Front", "Replace"}."Replace") -> ("Error out"=w410:errorcluster)  [unwired: 10 in, 1 out]
          }
          frame "Replace the existing database" {
            n132 = call-poly "General Enqueue Function - Data Logger.vi"("QRef in"=w411, "Array of Messages"=T13[] [{"state"=enum."Replace Database", "data"=variant}, {"state"=enum."Idle", "data"=variant}], "Error in"=w414, "Mode"=enum16{"Back", "Front", "Replace"}."Replace") -> ("Error out"=w415:errorcluster)  [unwired: 10 in, 1 out]
          }
          frame "[Logged] Data Viewer" {
            n133 = call-poly "General Enqueue Function - Data Logger.vi"("QRef in"=w416, "Array of Messages"=T13[] [{"state"=enum."Logged File Viewer", "data"=variant}, {"state"=enum."Idle", "data"=variant}], "Error in"=w419, "Mode"=enum16{"Back", "Front", "Replace"}."Replace") -> ("Error out"=w420:errorcluster)  [unwired: 10 in, 1 out]
          }
          frame "Defrag Prompt TDMS file" {
            n134 = call-poly "General Enqueue Function - Data Logger.vi"("QRef in"=w421, "Array of Messages"=T13[] [{"state"=enum."Defrag Prompt File", "data"=variant}, {"state"=enum."Idle", "data"=variant}], "Error in"=w424, "Mode"=enum16{"Back", "Front", "Replace"}."Replace") -> ("Error out"=w425:errorcluster)  [unwired: 10 in, 1 out]
          }
          frame "View Prompt TDMS file" {
            n135 = call-poly "General Enqueue Function - Data Logger.vi"("QRef in"=w426, "Array of Messages"=T13[] [{"state"=enum."View Prompt File", "data"=variant}, {"state"=enum."Idle", "data"=variant}], "Error in"=w429, "Mode"=enum16{"Back", "Front", "Replace"}."Replace") -> ("Error out"=w430:errorcluster)  [unwired: 10 in, 1 out]
          }
          frame "Create missing database" {
            n136 = call-poly "General Enqueue Function - Data Logger.vi"("QRef in"=w431, "Array of Messages"=T13[] [{"state"=enum."Create Database", "data"=variant}, {"state"=enum."Idle", "data"=variant}], "Error in"=w434, "Mode"=enum16{"Back", "Front", "Replace"}."Replace") -> ("Error out"=w435:errorcluster)  [unwired: 10 in, 1 out]
          }
          frame "Save Configuration" {
            n137 = To Variant(anything=enum16{"App", "User"}."User") -> (Variant=w440:variant)
            n138 = Bundle By Name(cluster=T13 {"state"=enum."Save to config file", "data"=variant} ("Q1 Message"), "data"=w440) -> (w436:T13)
            n139 = Build Array(w436, T13 {"state"=enum."Idle", "data"=variant} ("Q1 Message")) -> (w438:T13[])
            n140 = call-poly "General Enqueue Function - Data Logger.vi"("QRef in"=w442, "Array of Messages"=w438, "Error in"=w444, "Mode"=enum16{"Back", "Front", "Replace"}."Replace") -> ("Error out"=w445:errorcluster)  [unwired: 10 in, 1 out]
          }
          frame "Load Configuration" {
            n141 = To Variant(anything=enum16{"App", "User"}."User") -> (Variant=w450:variant)
            n142 = Bundle By Name(cluster=T13 {"state"=enum."Open from config file", "data"=variant} ("Q1 Message"), "data"=w450) -> (w446:T13)
            n143 = Build Array(w446, T13 {"state"=enum."Idle", "data"=variant} ("Q1 Message")) -> (w448:T13[])
            n144 = call-poly "General Enqueue Function - Data Logger.vi"("QRef in"=w452, "Array of Messages"=w448, "Error in"=w454, "Mode"=enum16{"Back", "Front", "Replace"}."Replace") -> ("Error out"=w455:errorcluster)  [unwired: 10 in, 1 out]
          }
          frame "HTML" {
            n145 = call "Data logger Default Paths.vi"("Path Type"=T12."Help HTML") -> ("Path"=w457:path)  [unwired: 4 in]
            n146 = Control Online Help(1:w459, 2:w457, 4:enum16{"Contents", "Key", "Close"}."Contents" ("Operation")) -> (0:w458:errorcluster)  [unwired: 1 in]
          }
          frame "Excel Template" {
            n147 = call "Data logger Default Paths.vi"("Path Type"=T12."Excel Template") -> ("Path"=w467:path)  [unwired: 4 in]
            n148 = call <vilib>:"New Report.vi"("window state (normal)"=T15."maximized", "report type"=T14."Excel", "template (empty)"=w467, "error in (no error)"=w462) -> ("report out"=w466:refnum<class "NI_report.lvclass">, "error out"=w465:errorcluster)  [unwired: 10 in]
            n149 = call-dynamic "Dispose Report.vi"("report in"=w466, "error in (no error)"=w465, "close report? (T)"=FALSE) -> ("error out"=w463:errorcluster)  [unwired: 12 in]
          }
          frame "MS Word doc" {
            n150 = call "Data logger Default Paths.vi"("Path Type"=T12."Help Word") -> ("Path"=w472:path)  [unwired: 4 in]
            n151 = call <vilib>:"New Report.vi"("window state (normal)"=T15."maximized", "report type"=T14."Word", "template (empty)"=w472, "error in (no error)"=w474) -> ("report out"=w476:refnum<class "NI_report.lvclass">, "error out"=w475:errorcluster)  [unwired: 10 in]
            n152 = call-dynamic "Dispose Report.vi"("report in"=w476, "error in (no error)"=w475, "close report? (T)"=FALSE) -> ("error out"=w471:errorcluster)  [unwired: 12 in]
          }
          frame "CSV Template" {
            n153 = call "Data logger Default Paths.vi"("Path Type"=T12."CSV Template") -> ("Path"=w482:path)  [unwired: 4 in]
            n154 = call "open in notepad.vi"("error in (no error)"=w480, "Path"=w482) -> ("error out"=w481:errorcluster)  [unwired: 9 in]
          }
          frame "Tray" {
            n155 = global read "Data Logger Global Variable.vi" "System Tray"() -> (w485:enum16{"Enabled", "Disabled"})
            n156 = case shown="\"Disabled\"" w485 {
              tunnel: [enum16{"Enabled", "Disabled"}."Disabled" ("System Tray") enum16{"Enabled", "Disabled"}."Enabled" ("System Tray")] -> w484
              tunnel: ["System Tray: Disabled" "System Tray: Enabled"] -> w489
              frame "Enabled", Default {
              }
              frame "Disabled" {
              }
            }
            n157 = global write "Data Logger Global Variable.vi" "System Tray"(w484) -> ()
            n158 = Set Menu Item Info(7:w486, 8:w488, 10:w489, 11:w483) -> (0:w487:errorcluster)  [unwired: 3 in, 1 out]
          }
          frame "Display 0" {
            n159 = global read "Data Logger Global Variable.vi" "Active Display"() -> (w502:u16)
            n160 = flat-sequence {
              tunnel: w502 -> [w506]
              tunnel: [u16 0 ("Active Display")] -> w501
              tunnel: [w506] -> w503
              frame #0 {
              }
            }
            n161 = global write "Data Logger Global Variable.vi" "Active Display"(w501) -> ()
            n162 = global read "Data Logger Global Variable.vi" "FP Bounds"() -> (w500:T2)
            n163 = global read "Data Logger Global Variable.vi" "Pane Origin"() -> (w499:T5[])
            n164 = call "Display on Menu - Action.vi"("Item Tag"=w494, "Previous Active Display"=w503, "Active Display"=w501, "error in"=w496, "MenuRef"=w497, "FP Bounds"=w500, "VI Ref"=w498) -> ("error out"=w504:errorcluster, "VI Ref"=w505:refnum<vi>)  [unwired: 3 in]
            n165 = call "Set Pane Origin.vi"("error in"=w504, "Pane Origin"=w499, "VI Ref"=w505) -> ("error out"=w495:errorcluster)  [unwired: 7 in, 1 out]
          }
          frame "Display 1" {
            n166 = global read "Data Logger Global Variable.vi" "Active Display"() -> (w516:u16)
            n167 = flat-sequence {
              tunnel: w516 -> [w520]
              tunnel: [u16 1 ("Active Display")] -> w515
              tunnel: [w520] -> w517
              frame #0 {
              }
            }
            n168 = global write "Data Logger Global Variable.vi" "Active Display"(w515) -> ()
            n169 = global read "Data Logger Global Variable.vi" "FP Bounds"() -> (w514:T2)
            n170 = global read "Data Logger Global Variable.vi" "Pane Origin"() -> (w513:T5[])
            n171 = call "Display on Menu - Action.vi"("Item Tag"=w508, "Previous Active Display"=w517, "Active Display"=w515, "error in"=w510, "MenuRef"=w511, "FP Bounds"=w514, "VI Ref"=w512) -> ("error out"=w518:errorcluster, "VI Ref"=w519:refnum<vi>)  [unwired: 3 in]
            n172 = call "Set Pane Origin.vi"("error in"=w518, "Pane Origin"=w513, "VI Ref"=w519) -> ("error out"=w509:errorcluster)  [unwired: 7 in, 1 out]
          }
          frame "Display 2" {
            n173 = global read "Data Logger Global Variable.vi" "Active Display"() -> (w530:u16)
            n174 = flat-sequence {
              tunnel: w530 -> [w534]
              tunnel: [u16 2 ("Active Display")] -> w529
              tunnel: [w534] -> w531
              frame #0 {
              }
            }
            n175 = global write "Data Logger Global Variable.vi" "Active Display"(w529) -> ()
            n176 = global read "Data Logger Global Variable.vi" "FP Bounds"() -> (w528:T2)
            n177 = global read "Data Logger Global Variable.vi" "Pane Origin"() -> (w527:T5[])
            n178 = call "Display on Menu - Action.vi"("Item Tag"=w522, "Previous Active Display"=w531, "Active Display"=w529, "error in"=w524, "MenuRef"=w525, "FP Bounds"=w528, "VI Ref"=w526) -> ("error out"=w532:errorcluster, "VI Ref"=w533:refnum<vi>)  [unwired: 3 in]
            n179 = call "Set Pane Origin.vi"("error in"=w532, "Pane Origin"=w527, "VI Ref"=w533) -> ("error out"=w523:errorcluster)  [unwired: 7 in, 1 out]
          }
          frame "Display 3" {
            n180 = global read "Data Logger Global Variable.vi" "Active Display"() -> (w544:u16)
            n181 = flat-sequence {
              tunnel: w544 -> [w548]
              tunnel: [u16 3 ("Active Display")] -> w543
              tunnel: [w548] -> w545
              frame #0 {
              }
            }
            n182 = global write "Data Logger Global Variable.vi" "Active Display"(w543) -> ()
            n183 = global read "Data Logger Global Variable.vi" "FP Bounds"() -> (w542:T2)
            n184 = global read "Data Logger Global Variable.vi" "Pane Origin"() -> (w541:T5[])
            n185 = call "Display on Menu - Action.vi"("Item Tag"=w536, "Previous Active Display"=w545, "Active Display"=w543, "error in"=w538, "MenuRef"=w539, "FP Bounds"=w542, "VI Ref"=w540) -> ("error out"=w546:errorcluster, "VI Ref"=w547:refnum<vi>)  [unwired: 3 in]
            n186 = call "Set Pane Origin.vi"("error in"=w546, "Pane Origin"=w541, "VI Ref"=w547) -> ("error out"=w537:errorcluster)  [unwired: 7 in, 1 out]
          }
          frame "Data Viewer" {
            # "Running Data Viewer from this runtime"
            n187 = call "Data logger Default Paths.vi"("Path Type"=T16."Data Viewer") -> ("Path"=w550:path)  [unwired: 4 in]
            n188 = Open VI Reference(vi path=w550, error in (no error)=w553) -> (vi reference=w556:refnum<vi>, error out=w558:errorcluster)  [unwired: 4 in]
            n189 = property class="VI"(reference=w556, error in=w558, "Front Panel Window:Open"=TRUE) -> (reference out=w555:refnum<vi>, error out=w557:errorcluster)
            n190 = invoke class="VI" method="Run VI"(reference=w555, error in=w557, "Wait until done"=FALSE, "Auto Dispose Ref"=TRUE) -> (error out=w552:errorcluster)  [unwired: 1 in, 4 out]
          }
        }
      }
      event "Exit Button": Value Change {
        n191 = event-data() -> ()  [unwired: 1 in, 2 out]
        n192 = To Variant(anything=enum16{"App", "User"}."App") -> (Variant=w572:variant)
        n193 = Bundle By Name(cluster=T13 {"state"=enum."Save to config file", "data"=variant} ("Q1 Message"), "data"=w572) -> (w570:T13)
        n194 = Build Array(w570, T13 {"state"=enum."Exit", "data"=variant} ("Q1 Message")) -> (w569:T13[])
        n195 = call-poly "General Enqueue Function - Data Logger.vi"("QRef in"=w575, "Array of Messages"=w569, "Error in"=w576, "Mode"=enum16{"Back", "Front", "Replace"}."Replace") -> ("QRef out"=w567:refnum<queue>, "Error out"=w566:errorcluster)  [unwired: 10 in]
        n196 = call-poly "General Enqueue Function - Data Logger.vi"("QRef in"=w563, "Array of Messages"=T13[] [{"state"=enum."Exit", "data"=variant}], "Error in"=w566) -> ("QRef out"=w562:refnum<queue>, "Error out"=w565:errorcluster)  [unwired: 11 in]
      }
      event "Record Button": Value Change {
        n197 = event-data() -> ()  [unwired: 1 in, 6 out]
        n198 = call-poly "General Enqueue Function - Data Logger.vi"("QRef in"=w585, "Array of Messages"=T13[] [{"state"=enum."Preparation 1", "data"=variant}, {"state"=enum."Preparation 2", "data"=variant}, {"state"=enum."Preparation 3", "data"=variant}, {"state"=enum."Preparation 4", "data"=variant}, {"state"=enum."Record", "data"=variant}], "Error in"=w580, "Mode"=enum16{"Back", "Front", "Replace"}."Replace") -> ("QRef out"=w586:refnum<queue>, "Error out"=w584:errorcluster)  [unwired: 10 in]
      }
      event "Stop Button": Value Change {
        n199 = event-data() -> ()  [unwired: 1 in, 6 out]
        n200 = call "Enqueue Q2.vi"("Q1 Message"=T13 {"state"=enum."Stop recording", "data"=variant}, "error in (no error)"=w590, "Queue Ref"=w593) -> ("error out"=w594:errorcluster)  [unwired: 5 in, 3 out]
      }
      event "Initialize": Value Change {
        n201 = event-data() -> ()  [unwired: 1 in, 6 out]
        n202 = control-ref of="Initialize"() -> (w600:refnum<vi>)
        n203 = property class="Bool"(reference=w600, error in=w602, "Blinking"=FALSE) -> (error out=w601:errorcluster)  [unwired: 1 out]
        n204 = call-poly "General Enqueue Function - Data Logger.vi"("QRef in"=w604, "Array of Messages"=T13[] [{"state"=enum."initialize 4", "data"=variant}, {"state"=enum."initialize 5", "data"=variant}, {"state"=enum."initialize 6", "data"=variant}, {"state"=enum."initialize 7", "data"=variant}, {"state"=enum."Idle", "data"=variant}], "Error in"=w601, "Mode"=enum16{"Back", "Front", "Replace"}."Replace") -> ("QRef out"=w605:refnum<queue>, "Error out"=w607:errorcluster)  [unwired: 10 in]
      }
      event "View": Value Change {
        n205 = event-data() -> ()  [unwired: 1 in, 6 out]
        n206 = Enqueue Element(queue=w613, element=T13 {"state"=enum."View", "data"=variant} ("Q1 Message"), error in (no error)=w612) -> (queue out=w616:refnum<queue>, error out=w614:errorcluster)  [unwired: 1 in, 1 out]
      }
      event "Deployed Libraries": Value Change {
        n207 = event-data() -> ()  [unwired: 1 in, 6 out]
        n208 = property on="Select All" class="Bool (strict)"(error in=w621, "Val(Sgnl)"=FALSE ("Value (Signaling)")) -> (error out=w620:errorcluster)  [unwired: 1 in, 1 out]
        n209 = property on="Variables" class="LstBox (strict)"(error in=w620, "Item Names"=string[] [], "Value"=i32[] [0] ("Variables")) -> (error out=w624:errorcluster)  [unwired: 1 in, 1 out]
        n210 = call-poly "General Enqueue Function - Data Logger.vi"("QRef in"=w625, "Array of Messages"=T13[] [{"state"=enum."initialize 6", "data"=variant}, {"state"=enum."initialize 7", "data"=variant}, {"state"=enum."Idle", "data"=variant}], "Error in"=w624, "Mode"=enum16{"Back", "Front", "Replace"}."Replace") -> ("QRef out"=w627:refnum<queue>, "Error out"=w628:errorcluster)  [unwired: 10 in]
      }
      event "create database": Value Change {
        n211 = event-data() -> ()  [unwired: 1 in, 6 out]
        n212 = call-poly "General Enqueue Function - Data Logger.vi"("QRef in"=w637, "Array of Messages"=T13[] [{"state"=enum."Create Database", "data"=variant}, {"state"=enum."Idle", "data"=variant}], "Error in"=w636) -> ("QRef out"=w638:refnum<queue>, "Error out"=w635:errorcluster)  [unwired: 11 in]
      }
      event "Add date/time to file name", "File Name": Value Change {
        n213 = event-data() -> ()  [unwired: 1 in, 6 out]
        n214 = control-ref of="Initialize"() -> (w645:refnum<vi>)
        n215 = property class="Bool"(reference=w645, error in=w646, "Blinking"=TRUE) -> (error out=w643:errorcluster)  [unwired: 1 out]
      }
      event "Folder Setting": Value Change {
        n216 = event-data() -> ()  [unwired: 1 in, 6 out]
        n217 = call-poly "General Enqueue Function - Data Logger.vi"("QRef in"=w652, "Q1 Message"=T13 {"state"=enum."Update folder setting", "data"=variant}, "Error in"=w650) -> ("QRef out"=w651:refnum<queue>, "Error out"=w653:errorcluster)  [unwired: 11 in]
      }
      event "Preference": Value Change {
        n218 = event-data() -> ()  [unwired: 1 in, 6 out]
        n219 = call-poly "General Enqueue Function - Data Logger.vi"("QRef in"=w660, "Q1 Message"=T13 {"state"=enum."Update Preference", "data"=variant}, "Error in"=w658) -> ("QRef out"=w659:refnum<queue>, "Error out"=w661:errorcluster)  [unwired: 11 in]
      }
      event "TDMS Properties": Value Change {
        n220 = event-data() -> ()  [unwired: 1 in, 3 out]
        n221 = call-poly "General Enqueue Function - Data Logger.vi"("QRef in"=w668, "Q1 Message"=T13 {"state"=enum."Update TDMS properties", "data"=variant}, "Error in"=w666) -> ("QRef out"=w667:refnum<queue>, "Error out"=w669:errorcluster)  [unwired: 11 in]
      }
      event "Select All": Value Change {
        n222 = event-data() -> ("NewVal"=w675:bool)  [unwired: 1 in, 1 out]
        n223 = case shown="True" w675 {
          tunnel: w674 -> [w681 w687]
          tunnel: [w680 w684] -> w673
          frame False {
            n224 = property on="Variables" class="LstBox (strict)"(error in=w681, "Val(Sgnl)"=i32[] [0] ("Value (Signaling)")) -> (error out=w680:errorcluster)  [unwired: 1 in, 1 out]
          }
          frame True {
            n225 = property on="Variables" class="LstBox (strict)"(error in=w687) -> (error out=w685:errorcluster, "Item Names"=w683:string[])  [unwired: 1 in, 1 out]
            n226 = Array Size(array=w683) -> (size(s)=w682:i32)
            n227 = for {
              N: w682 -> [_]
              tunnel: [w688] -> w686 mode=indexing
              i -> [w688]
            }
            n228 = property on="Variables" class="LstBox (strict)"(error in=w685, "Val(Sgnl)"=w686) -> (error out=w684:errorcluster)  [unwired: 1 in, 1 out]
          }
        }
      }
      event "Variables": Mouse Down; "Variables": Key Down {
        n229 = event-data() -> ("CtlRef"=w697:refnum<vi>)  [unwired: 1 in, 3 out]
        n230 = property class="LstBox (strict)"(reference=w697, error in=w690) -> (error out=w691:errorcluster, "Item Names"=w696:string[], "Value"=w695:i32[])  [unwired: 1 out]
        n231 = Array Size(array=w696) -> (size(s)=w693:i32)
        n232 = Array Size(array=w695) -> (size(s)=w694:i32)
        n233 = Not Equal?(x=w693, y=w694) -> (x != y?=w692:bool)
        n234 = case shown="False" w692 {
          tunnel: w691 -> [w702 w705]
          tunnel: [w702 w704] -> w698
          frame False {
          }
          frame True {
            n235 = property on="Select All" class="Bool (strict)"(error in=w705, "Value"=FALSE ("Select All")) -> (error out=w704:errorcluster)  [unwired: 1 in, 1 out]
          }
        }
      }
    }
    n236 = call "Data Logger Error Handling.vi"("error in"=w112, "Enum"=enum16{"Main", "Event", "Config"}."Event") -> ("error out"=w111:errorcluster)  [unwired: 7 in]
    n237 = Or(x=w111, y=w117) -> (x .or. y?=w116:bool)
  }
  n238 = while "Loop 1 - Data Logging Loop" {
    shift-right: [w719] -> _
    shift-left: w40 -> [w721]
    shift-right: [w706] -> w96
    shift-left: w62 -> [w722]
    shift-right: [w711] -> _
    shift-left: w81 -> [w712]
    tunnel: w68 -> [w710]
    stop <- w716 stop-if-true
    n239 = Dequeue Element(queue=w721, error in (no error)=w722) -> (queue out=w718:refnum<queue>, element=w720:T13, error out=w717:errorcluster)  [unwired: 1 in, 1 out]
    n240 = Unbundle By Name(w720) -> ("state"=w713:T1)
    "Application State" <- w713
    n241 = case shown="\"Defrag\"" w713 {
      tunnel: [w735 w782 w809 w838 w875 w902 w933 w960 w984 w985 w1065 w1082 w1114 w1155 w1165 w1177 w1202 w1225 w1239 w1259 w1283] -> w719
      tunnel: w718 -> [w736 w781 w810 w838 w875 w902 w933 w958 w984 w986 w1065 w1082 w1113 w1155 w1165 w1177 w1202 w1225 w1239 w1259 w1283]
      tunnel: w717 -> [w731 w778 w801 w841 w884 w923 w948 w951 w963 w995 w1058 w1080 w1109 w1159 w1164 w1176 w1206 w1221 w1236 w1248 w1276]
      tunnel: [w737 w783 w811 w837 w874 w901 w930 w959 w962 w997 w1051 w1080 w1112 w1132 w1164 w1171 w1201 w1224 w1238 w1251 w1282] -> w707
      tunnel: FALSE -> [w752 w784 w827 w842 w881 w921 w949 w956 w983 w999 w1064 w1091 w1123 w1158 w1163 w1180 w1210 w1233 w1246 w1261 w1297]
      tunnel: [w752 w784 w827 w842 w881 w921 w949 w956 w983 w999 w1064 w1091 w1123 w1158 w1162 w1180 w1210 w1233 w1246 w1261 w1297] -> w714
      tunnel: w712 -> [w751 w767 w826 w840 w879 w915 w945 w954 w982 w993 w1063 w1088 w1121 w1157 w1161 w1179 w1209 w1229 w1242 w1260 w1296]
      tunnel: [w749 w767 w826 w839 w878 w914 w945 w953 w982 w992 w1063 w1089 w1121 w1157 w1161 w1179 w1209 w1229 w1242 w1260 w1296] -> w711
      tunnel: w710 -> [_ _ _ _ _ _ _ _ _ _ _ _ w1115 _ _ _ _ _ _ _ _]
      tunnel: [w733 w766 w802 w836 w869 w895 w928 w952 w981 w998 w1062 w1081 w1102 w1154 w1160 w1175 w1200 w1223 w1237 w1258 w1281] -> w709
      tunnel: 100 ("timeout in ms (-1)") -> [w733 w766 w802 w836 w869 w895 w928 w952 w981 w998 w1062 w1081 w1102 w1154 w1160 w1175 w1200 w1223 w1237 w1258 w1281]
      frame "initialize 1", Default {
        w750 = string[] []
        # "Run at application startup"
        n242 = control-ref of="Exit Button"() -> (w738:refnum<vi>)
        n243 = control-ref of="Initialize"() -> (w739:refnum<vi>)
        n244 = control-ref of="Record Button"() -> (w740:refnum<vi>)
        n245 = control-ref of="Stop Button"() -> (w741:refnum<vi>)
        n246 = control-ref of="View"() -> (w742:refnum<vi>)
        n247 = control-ref of="Folder Setting"() -> (w727:refnum<vi>)
        n248 = control-ref of="Preference"() -> (w726:refnum<vi>)
        n249 = control-ref of="Add date/time to file name"() -> (w725:refnum<vi>)
        n250 = control-ref of="TDMS Properties"() -> (w724:refnum<vi>)
        n251 = Build Array(w727, w726, w725, w724) -> (w723:refnum<vi>[])
        n252 = Build Array(w738, w739, w740, w741, w742) -> (w743:refnum<vi>[])
        n253 = Bundle By Name(cluster=w751, "Bool Control Ref"=w743, "Selected Variables"=i32[] [], "DB availability for selected"=bool[] [], "DB path array"=path[] [] ("Database path array"), "TDMS file path"=path "C:/" ("appended path"), "TDMS ref"=refnum<k34> refnum ("tdms file out"), "Selected Variable Names"=w750, "Selected Variable URL"=w750, "Selected Variable Type"=w750, "Container Variable Name"=w750, "Container Variable URL"=w750, "Selected Library URL"=w750, "Library Name"=w750, "Library URL"=w750, "Seetings ref"=w723) -> (w749:T8)
        n254 = flat-sequence {
          tunnel: [FALSE] -> w732
          tunnel: w731 -> [w754]
          tunnel: [w754] -> w728
          tunnel: [u32 0 ("Clock Time")] -> w730
          frame #0 {
          }
        }
        n255 = global write "Recording Stop Watch.vi" "Start recording"(w732) -> ()
        n256 = global write "Recording Stop Watch.vi" "no message"(w732) -> ()
        n257 = global write "Recording Stop Watch.vi" "Clock Time"(w730) -> ()
        n258 = call "Data Logger Error Handling.vi"("error in"=w728) -> ("error out"=w729:errorcluster)  [unwired: 8 in]
        n259 = Enqueue Element(queue=w736, element=T13 {"state"=enum."initialize 2", "data"=variant} ("Q1 Message"), error in (no error)=w729) -> (queue out=w735:refnum<queue>, error out=w737:errorcluster)  [unwired: 1 in, 1 out]
      }
      frame "initialize 2" {
        w768 = FALSE ("Visible")
        n260 = control-ref of="Buffer size"() -> (w779:refnum<vi>)
        n261 = control-ref of="delimiter"() -> (w759:refnum<vi>)
        n262 = control-ref of="DB Type"() -> (w756:refnum<vi>)
        n263 = control-ref of="Description"() -> (w765:refnum<vi>)
        n264 = control-ref of="Author"() -> (w764:refnum<vi>)
        n265 = control-ref of="Title"() -> (w763:refnum<vi>)
        n266 = control-ref of="Server Name"() -> (w762:refnum<vi>)
        n267 = control-ref of="Invisible Libraries"() -> (w760:refnum<vi>)
        n268 = property class="DigNum (strict)"(reference=w779, error in=w778, "Visible"=w768) -> (error out=w777:errorcluster)  [unwired: 1 out]
        n269 = Build Array(w765, w764, w763, w762, w760, w759, w756) -> (w761:refnum<vi>[])
        n270 = control-ref of="database folder"() -> (w775:refnum<vi>)
        n271 = for {
          tunnel: w768 -> [w786]
          shift-right: [w787] -> w776
          shift-left: w777 -> [w788]
          tunnel: w761 -> [w785] mode=indexing
          n272 = property class="Ctl"(reference=w785, error in=w788, "Visible"=w786) -> (error out=w787:errorcluster)  [unwired: 1 out]
        }
        n273 = property class="Path"(reference=w775, error in=w776, "Visible"=w768) -> (error out=w774:errorcluster)  [unwired: 1 out]
        n274 = control-ref of="Folder to store TDMS file"() -> (w773:refnum<vi>)
        n275 = control-ref of="Sampling Period"() -> (w771:refnum<vi>)
        n276 = property class="Path"(reference=w773, error in=w774, "Visible"=w768) -> (error out=w772:errorcluster)  [unwired: 1 out]
        n277 = property class="DigNum (strict)"(reference=w771, error in=w772, "Visible"=w768) -> (error out=w769:errorcluster)  [unwired: 1 out]
        n278 = control-ref of="Auto Defrag"() -> (w770:refnum<vi>)
        n279 = property class="Bool (strict)"(reference=w770, error in=w769, "Visible"=w768) -> (error out=w757:errorcluster)  [unwired: 1 out]
        n280 = call "Data Logger Error Handling.vi"("error in"=w757) -> ("error out"=w758:errorcluster)  [unwired: 8 in]
        n281 = Enqueue Element(queue=w781, element=T13 {"state"=enum."initialize 3", "data"=variant} ("Q1 Message"), error in (no error)=w758) -> (queue out=w782:refnum<queue>, error out=w783:errorcluster)  [unwired: 1 in, 1 out]
      }
      frame "initialize 3" {
        w789 = T22."Enabled" ("Enable State")
        w812 = 2 ("length")
        # "Set Enable state of controls, clear list boxes"
        n282 = Unbundle By Name(w826) -> ("Seetings ref"=w790:refnum<vi>[], "Bool Control Ref"=w822:refnum<vi>[])
        n283 = property on="Registered file name" class="Str"(error in=w801, "Value"="") -> (error out=w800:errorcluster)  [unwired: 1 in, 1 out]
        n284 = Array Subset(array=w822, index=0, length=w812) -> (w824:refnum<vi>[])
        n285 = Array Subset(array=w822, index=w812, length=3) -> (w821:refnum<vi>[])
        n286 = call "Set Enable State Boolean.vi"("error in (no error)"=w800, "Enable State"=w789, "Boolean Ref Array"=w824) -> ("error out"=w792:errorcluster)  [unwired: 7 in, 1 out]
        n287 = control-ref of="Deployed Libraries"() -> (w818:refnum<vi>)
        n288 = control-ref of="Variables"() -> (w817:refnum<vi>)
        n289 = call "Set Enable State Boolean.vi"("error in (no error)"=w792, "Enable State"=w789, "Boolean Ref Array"=w790) -> ("error out"=w791:errorcluster)  [unwired: 7 in, 1 out]
        n290 = Build Array(w818, w817) -> (w816:refnum<vi>[])
        n291 = call "Set Enable State Boolean.vi"("error in (no error)"=w791, "Enable State"=T22."Disabled and Grayed Out", "Boolean Ref Array"=w821) -> ("error out"=w815:errorcluster)  [unwired: 7 in, 1 out]
        n292 = for {
          tunnel: w816 -> [w832] mode=indexing
          tunnel: string[] [] ("Item Names") -> [w830]
          shift-right: [w829] -> w813
          shift-left: w815 -> [w831]
          tunnel: string[] ["Deployed Libraries", "Variables"] ("Item Names") -> [w828] mode=indexing
          n293 = property class="LstBox (strict)"(reference=w832, error in=w831, "Item Names"=w830, "Caption.Text"=w828) -> (error out=w829:errorcluster)  [unwired: 1 out]
        }
        n294 = property on="Database Status" class="Str"(error in=w813, "Val(Sgnl)"="" ("Value (Signaling)")) -> (error out=w806:errorcluster)  [unwired: 1 in, 1 out]
        n295 = Current VI's Menubar() -> (w805:refnum<k9>)
        n296 = call "Set Menu Properties.vi"("menu reference"=w805, "Menu Tag"=string[] ["View", "Defrag", "Database"] ("item tags"), "enabled"=FALSE, "error in (no error)"=w806) -> ("error out"=w794:errorcluster)  [unwired: 7 in]
        n297 = property on="Select All" class="Bool (strict)"(error in=w794, "Value"=FALSE ("Select All")) -> (error out=w793:errorcluster)  [unwired: 1 in, 1 out]
        n298 = property on="Invisible Libraries" class="Arr (strict)"(error in=w793, "Val(Sgnl)"=string[] ["System", "NI_SSLConfiguration"] ("Value (Signaling)")) -> (error out=w797:errorcluster)  [unwired: 1 in, 1 out]
        n299 = call "Data Logger Error Handling.vi"("error in"=w797) -> ("error out"=w798:errorcluster)  [unwired: 8 in]
        n300 = Enqueue Element(queue=w810, element=T13 {"state"=enum."Idle", "data"=variant} ("Q1 Message"), error in (no error)=w798) -> (queue out=w809:refnum<queue>, error out=w811:errorcluster)  [unwired: 1 in, 1 out]
      }
      frame "initialize 4" {
        # "Build the TDMS file name and path"
        n301 = Equal?(x="File Name", y="") -> (x = y?=w834:bool)
        n302 = case shown="False" w834 {
          tunnel: "Add date/time to file name" -> [w854 _]
          tunnel: w841 -> [w849 _]
          tunnel: w840 -> [w848 w867]
          tunnel: [w846 w867] -> w839
          tunnel: [w845 errorcluster {"status"=TRUE, "code"=7021, "source"="Main Loop - Initialize 4"} ("error out")] -> w837
          tunnel: "File Name" -> [w844 _]
          frame False {
            n303 = case shown="False" w854 {
              tunnel: w844 -> [w859 w865]
              tunnel: [w859 w864] -> w850
              frame False {
              }
              frame True {
                n304 = Get Date/Time In Seconds() -> (seconds since 1Jan1904=w862:timestamp)
                n305 = Format Date/Time String(time format string (%c)="%Y.%m.%d_%H.%M.%S", seconds (now)=w862) -> (date/time string=w860:string)  [unwired: 1 in]
                n306 = Concatenate Strings(w865, " - " ("string"), w860) -> (w864:string)
              }
            }
            "Registered file name" <- w850
            n307 = Concatenate Strings(w850, ".tdms" ("string")) -> (w852:string)
            n308 = Build Path(base path="Folder to store TDMS file", name or relative path=w852) -> (appended path=w847:path)
            n309 = flat-sequence {
              tunnel: w849 -> [w858]
              tunnel: [w858] -> w845
              tunnel: w848 -> [w857]
              tunnel: w847 -> [w856]
              tunnel: [w855] -> w846
              frame #0 {
                n310 = Bundle By Name(cluster=w857, "TDMS file path"=w856) -> (w855:T8)
              }
            }
          }
          frame True {
          }
        }
      }
      frame "initialize 5" {
        # "Get the deployed Processes Names and URLs"
        n311 = call "Get Process List.vi"("Invisible Libraries"="Invisible Libraries", "Error In"=w884, "Remove Library"=TRUE ("Remove \"System\" library"), "Server Name"="Server Name") -> ("Error Out"=w882:errorcluster, "Libraries"=w883:T24)  [unwired: 5 in, 1 out]
        n312 = Unbundle By Name(w883) -> ("library URL"=w877:string[], "Library Name"=w876:string[])
        n313 = Bundle By Name(cluster=w879, "Library URL"=w877, "Library Name"=w876) -> (w878:T8)
        n314 = Array Size(array=w876) -> (size(s)=w872:i32)
        n315 = call "Make Caption.vi"("Mode"=enum16{"Libraries", "Variables"}."Libraries", "size(s)"=w872) -> ("Caption"=w870:string)  [unwired: 9 in]
        n316 = property on="Deployed Libraries" class="LstBox (strict)"(error in=w882, "Item Names"=w876, "Top Row"=0, "Caption.Text"=w870) -> (error out=w874:errorcluster)  [unwired: 1 in, 1 out]
      }
      frame "initialize 6" {
        # "Get the variable names and URLs for the selected Deployed Library(process), and display\nLooks for database files, if not found or found more than one, it is reported to user"
        n317 = Unbundle By Name(w915) -> ("Library Name"=w908:string[], "Library URL"=w909:string[])
        n318 = control-ref of="Record Button"() -> (w917:refnum<vi>)
        n319 = control-ref of="create database"() -> (w916:refnum<vi>)
        n320 = control-ref of="Database Status"() -> (w911:refnum<vi>)
        n321 = Build Array(w916, w917) -> (w912:refnum<vi>[])
        n322 = call "Get Variable List.vi"("Error In"=w923, "Selected Libraries"="Deployed Libraries", "library URL"=w909, "library Name"=w908) -> ("Error Out"=w920:errorcluster, "Selected Library Names"=w924:string[], "Selected Library URLs"=w905:string[], "Variable"=w922:T25)  [unwired: 4 in]
        n323 = call "Build Database Path.vi"("DB Type"="DB Type", "Error In"=w920, "Selected Library Names"=w924, "Folder containing database files"="database folder") -> ("Error Out"=w910:errorcluster, "Database not available for at least one?"=w913:bool, "Database Availability for selected libraries"=w903:bool[], "Database path array for selected libraries"=w904:path[], "More than one database?"=w887:bool[])  [unwired: 3 in]
        n324 = Unbundle By Name(w922) -> ("Variable Name"=w907:string[], "Variable URL"=w906:string[])
        n325 = Current VI's Menubar() -> (w896:refnum<k9>)
        n326 = Search 1D Array(1D array=w887, element=TRUE, start index (0)=0) -> (index of element=w890:i32)
        n327 = call "Database Check.vi"("Menu ref"=w896, "error in (no error)"=w910, "Database status ref"=w911, "Array ref in"=w912, "Database not available for at least one?"=w913) -> ("error out"=w894:errorcluster)  [unwired: 6 in]
        n328 = Not Equal?(x=w890, y=-1) -> (x != y?=w892:bool)
        n329 = call "Display Message to User3"("error in (no error)"=w894, "Enable"=w892) -> ("error out"=w893:errorcluster)  [unwired: 8 in, 1 out]
        n330 = Array Size(array=w907) -> (size(s)=w897:i32)
        n331 = call "Make Caption.vi"("Mode"=enum16{"Libraries", "Variables"}."Variables", "size(s)"=w897) -> ("Caption"=w899:string)  [unwired: 9 in]
        n332 = Bundle By Name(cluster=w915, "Container Variable Name"=w907, "Container Variable URL"=w906, "Selected Library URL"=w905, "DB path array"=w904, "DB availability for selected"=w903) -> (w914:T8)
        n333 = property on="Variables" class="LstBox (strict)"(error in=w893, "Item Names"=w907, "Top Row"=0 ("Active Row:Active Row Number"), "Caption.Text"=w899) -> (error out=w901:errorcluster)  [unwired: 1 in, 1 out]
      }
      frame "initialize 7" {
        w926 = T22."Enabled" ("Disabled")
        # "Set Enable state of controls and menu"
        n334 = Unbundle By Name(w945) -> ("Bool Control Ref"=w937:refnum<vi>[])
        n335 = Index Array(array=w937, index #1=1 ("index"), index #2=0 ("index"), index #3=4 ("index")) -> (element #1=w941:refnum<vi>, element #2=w940:refnum<vi>, element #3=w939:refnum<vi>)
        n336 = Index Array(array=w937, index=3) -> (element=w936:refnum<vi>)
        n337 = Build Array(w941, w940, w939) -> (w938:refnum<vi>[])
        n338 = Build Array(w936) -> (w946:refnum<vi>[])
        n339 = call "Set Enable State Boolean.vi"("error in (no error)"=w948, "Enable State"=w926, "Boolean Ref Array"=w938) -> ("error out"=w947:errorcluster)  [unwired: 7 in, 1 out]
        n340 = call "Set Enable State Boolean.vi"("error in (no error)"=w947, "Enable State"=T22."Disabled and Grayed Out" ("Disabled"), "Boolean Ref Array"=w946) -> ("error out"=w927:errorcluster)  [unwired: 7 in, 1 out]
        n341 = property on="File Name" class="Str"(error in=w927, "DisabledEnum"=w926) -> (error out=w925:errorcluster)  [unwired: 1 in, 1 out]
        n342 = Current VI's Menubar() -> (w931:refnum<k9>)
        n343 = call "Set Menu Properties.vi"("menu reference"=w931, "Menu Tag"=string[] ["View", "Defrag", "Database"] ("item tags"), "enabled"=TRUE, "error in (no error)"=w925) -> ("error out"=w930:errorcluster)  [unwired: 7 in]
      }
      frame "Idle" {
        n344 = Bundle By Name(cluster=w954, "Selected Variables"="Variables") -> (w953:T8)
        n345 = call "Data Logger Error Handling.vi"("error in"=w951) -> ("error out"=w950:errorcluster)  [unwired: 8 in]
        n346 = Enqueue Element(queue=w958, element=T13 {"state"=enum."Idle", "data"=variant} ("Q1 Message"), error in (no error)=w950) -> (queue out=w960:refnum<queue>, error out=w959:errorcluster)  [unwired: 1 in, 1 out]
      }
      frame "Preparation 1" {
        w961 = T22."Disabled and Grayed Out" ("Disabled")
        n347 = control-ref of="TDMS Properties"() -> (w980:refnum<vi>)
        n348 = control-ref of="Add date/time to file name"() -> (w974:refnum<vi>)
        n349 = control-ref of="Initialize"() -> (w966:refnum<vi>)
        n350 = control-ref of="Record Button"() -> (w964:refnum<vi>)
        n351 = control-ref of="Exit Button"() -> (w965:refnum<vi>)
        n352 = control-ref of="Folder Setting"() -> (w972:refnum<vi>)
        n353 = control-ref of="Preference"() -> (w973:refnum<vi>)
        n354 = control-ref of="View"() -> (w971:refnum<vi>)
        n355 = Build Array(w966, w964, w965, w971, w972, w973, w974, w980) -> (w969:refnum<vi>[])
        n356 = call "Set Enable State Boolean.vi"("error in (no error)"=w963, "Enable State"=w961, "Boolean Ref Array"=w969) -> ("error out"=w970:errorcluster)  [unwired: 7 in, 1 out]
        n357 = control-ref of="Stop Button"() -> (w968:refnum<vi>)
        n358 = property class="Bool"(reference=w968, error in=w970, "DisabledEnum"=T22."Enabled" ("Disabled")) -> (error out=w975:errorcluster)  [unwired: 1 out]
        n359 = property on="File Name" class="Str"(error in=w975, "DisabledEnum"=w961) -> (error out=w976:errorcluster)  [unwired: 1 in, 1 out]
        n360 = Current VI's Menubar() -> (w979:refnum<k9>)
        n361 = call "Set Menu Properties.vi"("menu reference"=w979, "Menu Tag"=string[] ["View", "Defrag", "Folder Setting", "Preference", "Database", "Log File Properties"] ("item tags"), "enabled"=FALSE, "error in (no error)"=w976) -> ("error out"=w962:errorcluster)  [unwired: 7 in]
      }
      frame "Preparation 2" {
        # "Not a good solution"
        # "Make ref to TDMS file and Add TDMS root Properties"
        n362 = Unbundle By Name(w993) -> ("TDMS file path"=w996:path)
        n363 = call <vilib>:"Check if File or Folder Exists.vi"("error in (no error)"=w995, "path"=w996) -> ("error out"=w990:errorcluster, "file or folder exists?"=w987:bool, "dup path"=w991:path)  [unwired: 7 in]
        n364 = TDMS Open(8:w990, 10:T23."open or create" ("operation (0:open)"), 11:w991) -> (0:w989:errorcluster, 3:w988:refnum<k34>)  [unwired: 4 in]
        n365 = Bundle By Name(cluster=w993, "TDMS ref"=w988) -> (w992:T8)
        n366 = case shown="No Error" w989 {
          selector: w989 -> [w1011 _]
          tunnel: [w1013 w1044] -> w997
          tunnel: w988 -> [w1010 _]
          tunnel: w987 -> [w1005 _]
          tunnel: w986 -> [w1000 w1045]
          tunnel: [w1000 w1041] -> w985
          frame No Error {
            n367 = Build Array("Title", "Description", "Author") -> (w1014:string[])
            n368 = TDMS Set Properties(5:w1014, 7:string[] ["Title", "Description", "Author"], 8:w1011, 11:w1010) -> (0:w1007:errorcluster, 3:w1006:refnum<k34>)  [unwired: 2 in, 2 out]
            n369 = case shown="True" w1005 {
              tunnel: [w1023 w1030] -> w1004
              tunnel: [w1022 w1031] -> w1003
              tunnel: ["DateTime" ("property names") w1035] -> w1002
              tunnel: "Appendix_no" ("property names") -> [w1021 w1034]
              tunnel: i16 0 -> [w1020 w1038]
              tunnel: w1007 -> [w1018 w1028]
              tunnel: w1006 -> [w1019 w1027]
              frame False {
                n370 = TDMS Set Properties(5:w1020, 7:w1021, 8:w1018, 11:w1019) -> (0:w1022:errorcluster, 3:w1023:refnum<k34>)  [unwired: 2 in, 2 out]
              }
              frame True {
                n371 = TDMS Get Properties(5:w1038, 7:w1034, 8:w1028, 11:w1027) -> (0:w1036:errorcluster, 3:w1029:refnum<k34>, 4:w1037:i16)  [unwired: 2 in, 3 out]
                n372 = Increment(x=w1037) -> (x+1=w1033:i16)
                n373 = Format Into String(error in=w1036, w1033) -> (resulting string=w1025:string, error out=w1032:errorcluster)  [unwired: 2 in]
                n374 = TDMS Set Properties(5:w1033, 7:w1034, 8:w1032, 11:w1029) -> (0:w1031:errorcluster, 3:w1030:refnum<k34>)  [unwired: 2 in, 2 out]
                n375 = Concatenate Strings("DataTime_App_" ("property names"), w1025) -> (w1035:string)
              }
            }
            n376 = Get Date/Time In Seconds() -> (seconds since 1Jan1904=w1012:timestamp)
            n377 = TDMS Set Properties(5:w1012, 7:w1002, 8:w1003, 11:w1004) -> (0:w1013:errorcluster)  [unwired: 2 in, 3 out]
          }
          frame Error {
            # "if there is a problem with tdms creation"
            n378 = call "Data Logger Error Handling.vi"("error in"=errorcluster {"status"=TRUE, "code"=7100, "source"=""}) -> ("error out"=w1039:errorcluster)  [unwired: 8 in]
            n379 = call-poly "General Enqueue Function - Data Logger.vi"("QRef in"=w1045, "Array of Messages"=T13[] [{"state"=enum."initialize 3", "data"=variant}], "Error in"=w1039, "Mode"=enum16{"Back", "Front", "Replace"}."Replace") -> ("QRef out"=w1041:refnum<queue>, "Error out"=w1044:errorcluster)  [unwired: 10 in]
          }
        }
      }
      frame "Preparation 3" {
        n380 = control-ref of="Auto Defrag"() -> (w1061:refnum<vi>)
        n381 = property class="Bool (strict)"(reference=w1061, error in=w1058) -> (error out=w1059:errorcluster, "Value"=w1055:bool)  [unwired: 1 out]
        n382 = control-ref of="Buffer size"() -> (w1060:refnum<vi>)
        n383 = property class="DigNum (strict)"(reference=w1060, error in=w1059) -> (error out=w1052:errorcluster, "Value"=w1057:u32)  [unwired: 1 out]
        n384 = global read "Recording Stop Watch.vi" "no message"() -> (w1046:bool)
        n385 = Not(x=w1055) -> (.not. x?=w1053:bool)
        n386 = Less?(x=w1057, y=i64 50) -> (x < y?=w1054:bool)
        n387 = And(x=w1054, y=w1053) -> (x .and. y?=w1048:bool)
        n388 = Not(x=w1046) -> (.not. x?=w1047:bool)
        n389 = And(x=w1048, y=w1047) -> (x .and. y?=w1049:bool)
        n390 = case shown="True" w1049 {
          tunnel: w1052 -> [w1067 w1070]
          tunnel: [w1067 w1069] -> w1051
          tunnel: [w1066 w1068] -> w1050
          tunnel: w1046 -> [w1066 _]
          frame False {
          }
          frame True {
            n391 = call "Too smal buffer size"("error in (no error)"=w1070) -> ("Do not show this message."=w1068:bool, "error out"=w1069:errorcluster)  [unwired: 16 in, 1 out]
          }
        }
        n392 = global write "Recording Stop Watch.vi" "no message"(w1050) -> ()
      }
      frame "Preparation 4" {
        n393 = Unbundle By Name(w1088) -> ("Selected Variables"=w1085:i32[], "Container Variable Name"=w1084:string[], "Container Variable URL"=w1083:string[], "DB path array"=w1079:path[])
        n394 = call "Read Database.vi"("delimiter"="delimiter", "DB path array"=w1079) -> ("Array out"=w1077:string[][])  [unwired: 8 in, 1 out]
        n395 = for {
          tunnel: w1085 -> [w1095] mode=indexing
          tunnel: w1084 -> [w1099]
          tunnel: w1083 -> [w1097]
          tunnel: [w1098] -> w1087 mode=indexing
          tunnel: [w1096] -> w1086 mode=indexing
          tunnel: [w1095] -> w1090 mode=indexing
          n396 = Index Array(array=w1099, index=w1095) -> (element=w1098:string)
          n397 = Index Array(array=w1097, index=w1095) -> (element=w1096:string)
        }
        n398 = Index Array(array=w1077, index (col)=1 ("disabled index (col)")) -> (element=w1075:string[])  [unwired: 1 in]
        n399 = Delete From Array(array=w1075, length=1, index=0 ("length")) -> (array with subset deleted=w1072:string[])  [unwired: 1 out]
        n400 = for {
          tunnel: w1090 -> [w1093] mode=indexing
          tunnel: [w1094] -> w1071 mode=indexing
          tunnel: w1072 -> [w1092]
          n401 = Index Array(array=w1092, index=w1093) -> (element=w1094:string)
        }
        n402 = Bundle By Name(cluster=w1088, "Selected Variable Names"=w1087, "Selected Variable URL"=w1086, "Selected Variable Type"=w1071) -> (w1089:T8)
      }
      frame "Record" {
        n403 = Unbundle By Name(w1121) -> ("TDMS ref"=w1120:refnum<k34>, "Selected Variable URL"=w1119:string[], "Selected Variable Type"=w1118:string[], "Selected Variable Names"=w1117:string[])
        n404 = Tick Count (ms)() -> (millisecond timer value=w1107:u32)
        n405 = flat-sequence {
          tunnel: w1109 -> [w1129]
          tunnel: [w1129] -> w1108
          tunnel: w1107 -> [w1128]
          tunnel: TRUE -> [w1127]
          frame #0 {
            n406 = global write "Recording Stop Watch.vi" "Start recording"(w1127) -> ()
            n407 = global write "Recording Stop Watch.vi" "Clock Time"(w1128) -> ()
          }
        }
        n408 = Bundle("Sampling Period"="Sampling Period", "TDMS ref"=w1120, "Selected Variable URL"=w1119, "Selected Variable Type"=w1118, "Selected Variable Names"=w1117) -> (w1116:T26)  [unwired: 1 in]
        n409 = case shown="False" "Auto Defrag" {
          tunnel: [T13[] [{"state"=enum."Stop recording", "data"=variant}, {"state"=enum."Defrag", "data"=variant}, {"state"=enum."Idle", "data"=variant}] T13[] [{"state"=enum."Stop recording", "data"=variant}, {"state"=enum."Idle", "data"=variant}]] -> w1111
          frame True {
          }
          frame False {
          }
        }
        n410 = call "LoggingBlock.vi"("Buffer size"="Buffer size", "error in"=w1108, "Data In"=w1116, "Queue Ref"=w1115) -> ("error out"=w1105:errorcluster)  [unwired: 7 in]
        n411 = flat-sequence {
          tunnel: w1105 -> [w1126]
          tunnel: [w1126] -> w1101
          tunnel: FALSE -> [w1125]
          frame #0 {
            n412 = global write "Recording Stop Watch.vi" "Start recording"(w1125) -> ()
          }
        }
        n413 = call "Data Logger Error Handling.vi"("error in"=w1101) -> ("error out"=w1100:errorcluster)  [unwired: 8 in]
        n414 = call-poly "General Enqueue Function - Data Logger.vi"("QRef in"=w1113, "Array of Messages"=w1111, "Error in"=w1100, "Mode"=enum16{"Back", "Front", "Replace"}."Replace") -> ("QRef out"=w1114:refnum<queue>, "Error out"=w1112:errorcluster)  [unwired: 10 in]
      }
      frame "Stop recording" {
        n415 = control-ref of="TDMS Properties"() -> (w1153:refnum<vi>)
        n416 = control-ref of="Add date/time to file name"() -> (w1146:refnum<vi>)
        n417 = control-ref of="Folder Setting"() -> (w1144:refnum<vi>)
        n418 = control-ref of="Preference"() -> (w1145:refnum<vi>)
        n419 = control-ref of="View"() -> (w1143:refnum<vi>)
        n420 = control-ref of="Initialize"() -> (w1135:refnum<vi>)
        n421 = control-ref of="Exit Button"() -> (w1136:refnum<vi>)
        n422 = Unbundle By Name(w1157) -> ("TDMS ref"=w1156:refnum<k34>)
        n423 = Build Array(w1143, w1135, w1136, w1144, w1145, w1146, w1153) -> (w1142:refnum<vi>[])
        n424 = TDMS Close(8:w1159, 11:w1156) -> (0:w1134:errorcluster)  [unwired: 1 out]
        n425 = call "Set Enable State Boolean.vi"("error in (no error)"=w1134, "Enable State"=T22."Enabled" ("Disabled"), "Boolean Ref Array"=w1142) -> ("error out"=w1139:errorcluster)  [unwired: 7 in, 1 out]
        n426 = control-ref of="Record Button"() -> (w1137:refnum<vi>)
        n427 = control-ref of="Stop Button"() -> (w1138:refnum<vi>)
        n428 = Build Array(w1137, w1138) -> (w1140:refnum<vi>[])
        n429 = call "Set Enable State Boolean.vi"("error in (no error)"=w1139, "Enable State"=T22."Disabled and Grayed Out" ("Disabled"), "Boolean Ref Array"=w1140) -> ("error out"=w1147:errorcluster)  [unwired: 7 in, 1 out]
        n430 = property on="File Name" class="Str"(error in=w1147, "DisabledEnum"=T22."Enabled" ("Disabled")) -> (error out=w1150:errorcluster)  [unwired: 1 in, 1 out]
        n431 = Current VI's Menubar() -> (w1152:refnum<k9>)
        n432 = call "Set Menu Properties.vi"("menu reference"=w1152, "Menu Tag"=string[] ["View", "Defrag", "Folder Setting", "Preference", "Database", "Log File Properties"] ("item tags"), "enabled"=TRUE, "error in (no error)"=w1150) -> ("error out"=w1132:errorcluster)  [unwired: 7 in]
      }
      frame "Exit" {
        n433 = Not(x=w1163) -> (.not. x?=w1162:bool)
      }
      frame "Defrag" {
        n434 = Unbundle By Name(w1179) -> ("TDMS file path"=w1178:path)
        n435 = call "Defragment is in Progress.vi"("error in (no error)"=w1176) -> ("error out"=w1169:errorcluster, "This VI"=w1174:refnum<vi>)  [unwired: 9 in]
        n436 = call <vilib>:"Check if File or Folder Exists.vi"("error in (no error)"=w1169, "path"=w1178) -> ("error out"=w1181:errorcluster, "file or folder exists?"=w1183:bool, "dup path"=w1182:path)  [unwired: 7 in]
        n437 = case shown="True" w1183 {
          selector: w1183 -> [w1185 w1188]
          tunnel: w1182 -> [_ w1191]
          tunnel: w1181 -> [w1186 w1190]
          tunnel: [w1186 w1189] -> w1167
          tunnel: [w1185 w1188] -> w1172
          tunnel: w1174 -> [w1184 w1187]
          tunnel: [w1184 w1187] -> w1173
          frame False {
          }
          frame True {
            n438 = TDMS Defragment(4:w1190, 7:w1191) -> (0:w1189:errorcluster)
          }
        }
        n439 = Not(x=w1172) -> (.not. x?=w1170:bool)
        n440 = invoke class="VI" method="FP.Close"(reference=w1173, error in=w1169) -> (error out=w1166:errorcluster)  [unwired: 1 in, 2 out]
        n441 = Merge Errors(w1166, w1167) -> (w1168:errorcluster)
        n442 = call "Display Message to User2"("error in (no error)"=w1168, "Enable"=w1170) -> ("error out"=w1171:errorcluster)  [unwired: 8 in, 1 out]
      }
      frame "View" {
        # "Previously, index 0, 1, 4 became enabled."
        n443 = Unbundle By Name(w1209) -> ("Bool Control Ref"=w1203:refnum<vi>[], "TDMS file path"=w1208:path)
        n444 = call "Set Enable State Boolean.vi"("error in (no error)"=w1206, "Enable State"=T22."Disabled and Grayed Out" ("Disabled"), "Boolean Ref Array"=w1203) -> ("error out"=w1205:errorcluster, "Boolean Ref Array"=w1195:refnum<vi>[])  [unwired: 7 in]
        n445 = call <vilib>:"Check if File or Folder Exists.vi"("error in (no error)"=w1205, "path"=w1208) -> ("error out"=w1211:errorcluster, "file or folder exists?"=w1213:bool, "dup path"=w1212:path)  [unwired: 7 in]
        n446 = case shown="True" w1213 {
          selector: w1213 -> [w1214 w1216]
          tunnel: w1212 -> [_ w1219]
          tunnel: w1211 -> [w1215 w1218]
          tunnel: [w1215 w1217] -> w1198
          tunnel: [w1214 w1216] -> w1199
          frame False {
          }
          frame True {
            n447 = call <vilib>:"TDMS - File Viewer.vi"("error in (no error)"=w1218, "file path"=w1219) -> ("error out"=w1217:errorcluster)  [unwired: 4 in, 1 out]
          }
        }
        n448 = Not(x=w1199) -> (.not. x?=w1196:bool)
        n449 = call "Display Message to User"("error in (no error)"=w1198, "Enable"=w1196) -> ("error out"=w1197:errorcluster)  [unwired: 8 in, 1 out]
        n450 = Delete From Array(array=w1195, length=1, index=3) -> (array with subset deleted=w1192:refnum<vi>[])  [unwired: 1 out]
        n451 = call "Set Enable State Boolean.vi"("error in (no error)"=w1197, "Enable State"=T22."Enabled" ("Disabled"), "Boolean Ref Array"=w1192) -> ("error out"=w1201:errorcluster)  [unwired: 7 in, 1 out]
      }
      frame "Create Database" {
        # "Create DB for the selected deployed library"
        n452 = Unbundle By Name(w1229) -> ("Selected Library URL"=w1228:string[], "DB path array"=w1227:path[], "DB availability for selected"=w1226:bool[])
        n453 = property on="delimiter" class="Str"(error in=w1221) -> (error out=w1222:errorcluster, "Value"=w1220:string)  [unwired: 1 in, 1 out]
        n454 = property on="Deployed Libraries" class="LstBox (strict)"(error in=w1222) -> (error out=w1232:errorcluster, "Value"=w1231:i32[])  [unwired: 1 in, 1 out]
        n455 = call "CreateDatabase.vi"("delimiter"=w1220, "Error In"=w1232, "Database Availability"=w1226, "Database path array"=w1227, "Selected Library URLs"=w1228) -> ("Error Out"=w1230:errorcluster)  [unwired: 6 in]
        n456 = property on="Deployed Libraries" class="LstBox (strict)"(error in=w1230, "Val(Sgnl)"=w1231) -> (error out=w1224:errorcluster)  [unwired: 1 in, 1 out]
      }
      frame "Replace Database" {
        # "Create DB for the selected deployed library"
        n457 = Unbundle By Name(w1242) -> ("Selected Library URL"=w1241:string[], "DB path array"=w1240:path[])
        n458 = property on="delimiter" class="Str"(error in=w1236) -> (error out=w1235:errorcluster, "Value"=w1234:string)  [unwired: 1 in, 1 out]
        n459 = property on="Deployed Libraries" class="LstBox (strict)"(error in=w1235) -> (error out=w1245:errorcluster, "Value"=w1244:i32[])  [unwired: 1 in, 1 out]
        n460 = call "ReplaceDatabase.vi"("delimiter"=w1234, "Error In"=w1245, "Database path array"=w1240, "Selected Library URLs"=w1241) -> ("Error Out"=w1243:errorcluster)  [unwired: 7 in]
        n461 = property on="Deployed Libraries" class="LstBox (strict)"(error in=w1243, "Val(Sgnl)"=w1244) -> (error out=w1238:errorcluster)  [unwired: 1 in, 1 out]
      }
      frame "Defrag Prompt File" {
        n462 = control-ref of="Folder to store TDMS file"() -> (w1250:refnum<vi>)
        n463 = property class="Path"(reference=w1250, error in=w1248) -> (error out=w1247:errorcluster, "Value"=w1249:path)  [unwired: 1 out]
        n464 = call "File Dialog"("start path"=w1249, "prompt"="Select a TDMS file", "button label"="Defrag", "error in"=w1247, "pattern (all files)"="*.tdms") -> ("selected path"=w1252:path, "cancelled"=w1254:bool, "error out"=w1253:errorcluster)  [unwired: 7 in, 1 out]
        n465 = case shown="True" w1254 {
          tunnel: w1253 -> [w1267 w1269]
          tunnel: w1252 -> [w1265 _]
          tunnel: [w1262 w1268] -> w1251
          frame False {
            n466 = call "Defragment is in Progress.vi"("error in (no error)"=w1267) -> ("error out"=w1266:errorcluster, "This VI"=w1263:refnum<vi>)  [unwired: 9 in]
            n467 = TDMS Defragment(4:w1266, 7:w1265) -> (0:w1264:errorcluster)
            n468 = invoke class="VI" method="FP.Close"(reference=w1263, error in=w1264) -> (error out=w1262:errorcluster)  [unwired: 1 in, 2 out]
          }
          frame True {
            n469 = call <vilib>:"Clear Errors.vi"("error in (no error)"=w1269) -> ("error out"=w1268:errorcluster)  [unwired: 5 in, 1 out]
          }
        }
      }
      frame "View Prompt File" {
        n470 = control-ref of="Folder to store TDMS file"() -> (w1274:refnum<vi>)
        n471 = Unbundle By Name(w1296) -> ("Bool Control Ref"=w1292:refnum<vi>[])
        n472 = property class="Path"(reference=w1274, error in=w1276) -> (error out=w1275:errorcluster, "Value"=w1273:path)  [unwired: 1 out]
        n473 = call "Set Enable State Boolean.vi"("error in (no error)"=w1275, "Enable State"=T22."Disabled and Grayed Out" ("Disabled"), "Boolean Ref Array"=w1292) -> ("error out"=w1277:errorcluster, "Boolean Ref Array"=w1284:refnum<vi>[])  [unwired: 7 in]
        n474 = call "File Dialog2"("start path"=w1273, "prompt"="Select a TDMS file", "button label"="View", "error in"=w1277, "pattern (all files)"="*.tdms") -> ("selected path"=w1270:path, "cancelled"=w1271:bool, "error out"=w1272:errorcluster)  [unwired: 7 in, 1 out]
        n475 = case shown="False" w1271 {
          tunnel: [w1300 w1301] -> w1294
          tunnel: w1272 -> [w1299 w1302]
          tunnel: w1270 -> [w1298 _]
          frame False {
            n476 = call <vilib>:"TDMS - File Viewer.vi"("error in (no error)"=w1299, "file path"=w1298) -> ("error out"=w1300:errorcluster)  [unwired: 4 in, 1 out]
          }
          frame True {
            n477 = call <vilib>:"Clear Errors.vi"("error in (no error)"=w1302) -> ("error out"=w1301:errorcluster)  [unwired: 5 in, 1 out]
          }
        }
        n478 = Index Array(array=w1284, index #1=0 ("index"), index #2=1 ("index"), index #3=4 ("index")) -> (element #1=w1288:refnum<vi>, element #2=w1287:refnum<vi>, element #3=w1286:refnum<vi>)
        n479 = Build Array(w1288, w1287, w1286) -> (w1285:refnum<vi>[])
        n480 = call "Set Enable State Boolean.vi"("error in (no error)"=w1294, "Enable State"=T22."Enabled" ("Disabled"), "Boolean Ref Array"=w1285) -> ("error out"=w1282:errorcluster)  [unwired: 7 in, 1 out]
      }
    }
    n481 = Wait (ms)(milliseconds to wait=w709) -> ()  [unwired: 1 out]
    n482 = call "Data Logger Error Handling.vi"("error in"=w707) -> ("error out"=w706:errorcluster)  [unwired: 8 in]
    n483 = Or(x=w706, y=w714) -> (x .or. y?=w716:bool)
  }
  n484 = while "Loop 3 - Configuration Loop" {
    shift-right: [w1304] -> w61
    shift-left: w62 -> [w1318]
    tunnel: w63 -> [w1317]
    tunnel: w49 -> [w1307]
    tunnel: w40 -> [w1306]
    stop <- w1312 stop-if-true
    n485 = Dequeue Element(queue=w1317, error in (no error)=w1318) -> (queue out=w1315:refnum<queue>, element=w1313:T13, error out=w1316:errorcluster)  [unwired: 1 in, 1 out]
    n486 = Wait (ms)(milliseconds to wait=u32 100) -> ()  [unwired: 1 out]
    n487 = Unbundle By Name(w1313) -> ("state"=w1314:T1, "data"=w1308:variant)
    n488 = case shown="\"DB Type\"" w1314 {
      tunnel: w1316 -> [w1320 w1327 w1351 w1366 w1369 w1375 w1393 w1409 w1443 w1468 w1470]
      tunnel: w1315 -> [_ _ _ _ _ _ _ _ _ _ _]
      tunnel: [w1320 w1332 w1342 w1363 w1368 w1381 w1390 w1402 w1436 w1467 w1470] -> w1305
      tunnel: [w1319 w1333 w1352 w1367 w1374 w1384 w1398 w1410 w1444 w1469 w1471] -> w1311
      tunnel: FALSE -> [w1319 w1333 w1352 w1367 w1374 w1384 w1398 w1410 w1444 w1469 w1472]
      tunnel: w1308 -> [_ _ _ _ _ _ _ w1408 w1442 _ _]
      tunnel: w1307 -> [_ _ _ _ _ _ _ w1401 w1435 _ _]
      tunnel: w1306 -> [_ _ _ _ _ w1379 w1389 _ _ _ _]
      frame "Idle", Default {
      }
      frame "Update folder setting" {
        n489 = control-ref of="database folder"() -> (w1323:refnum<vi>)
        n490 = control-ref of="Folder to store TDMS file"() -> (w1324:refnum<vi>)
        n491 = property class="Path"(reference=w1324, error in=w1327) -> (error out=w1326:errorcluster, "Value"=w1321:path)  [unwired: 1 out]
        n492 = property class="Path"(reference=w1323, error in=w1326) -> (error out=w1325:errorcluster, "Value"=w1322:path)  [unwired: 1 out]
        n493 = call "Folder Setting.vi"("error in"=w1325, "Folder containing database files"=w1322, "Folder for saving log files"=w1321) -> ("error out"=w1330:errorcluster, "database folder"=w1329:path, "TDMS folder"=w1328:path)  [unwired: 6 in]
        n494 = property class="Path"(reference=w1323, error in=w1330, "Value"=w1329) -> (error out=w1331:errorcluster)  [unwired: 1 out]
        n495 = property class="Path"(reference=w1324, error in=w1331, "Value"=w1328) -> (error out=w1332:errorcluster)  [unwired: 1 out]
      }
      frame "Update Preference" {
        n496 = property on="Server Name" class="Str"(error in=w1351) -> (error out=w1350:errorcluster, "Value"=w1346:string)  [unwired: 1 in, 1 out]
        n497 = property on="Sampling Period" class="DigNum (strict)"(error in=w1350) -> (error out=w1349:errorcluster, "Value"=w1345:u32)  [unwired: 1 in, 1 out]
        n498 = property on="Buffer size" class="DigNum (strict)"(error in=w1349) -> (error out=w1348:errorcluster, "Value"=w1344:u32)  [unwired: 1 in, 1 out]
        n499 = property on="Auto Defrag" class="Bool (strict)"(error in=w1348) -> (error out=w1347:errorcluster, "Value"=w1343:bool)  [unwired: 1 in, 1 out]
        n500 = call "Preference.vi"("Auto Defrag"=w1343, "error in"=w1347, "Buffer size"=w1344, "Sampling Period"=w1345, "Server Name"=w1346) -> ("error out"=w1338:errorcluster, "Buffer size"=w1335:i64, "Sampling Period"=w1336:i64, "Server Name"=w1337:string, "Auto Defrag"=w1334:bool)  [unwired: 2 in]
        n501 = property on="Auto Defrag" class="Bool (strict)"(error in=w1338, "Value"=w1334) -> (error out=w1339:errorcluster)  [unwired: 1 in, 1 out]
        n502 = property on="Buffer size" class="DigNum (strict)"(error in=w1339, "Value"=w1335) -> (error out=w1340:errorcluster)  [unwired: 1 in, 1 out]
        n503 = property on="Sampling Period" class="DigNum (strict)"(error in=w1340, "Value"=w1336) -> (error out=w1341:errorcluster)  [unwired: 1 in, 1 out]
        n504 = property on="Server Name" class="Str"(error in=w1341, "Value"=w1337) -> (error out=w1342:errorcluster)  [unwired: 1 in, 1 out]
      }
      frame "Update TDMS properties" {
        n505 = property on="Author" class="Str"(error in=w1366) -> (error out=w1365:errorcluster, "Value"=w1357:string)  [unwired: 1 in, 1 out]
        n506 = property on="Description" class="Str"(error in=w1365) -> (error out=w1364:errorcluster, "Value"=w1358:string)  [unwired: 1 in, 1 out]
        n507 = property on="Title" class="Str"(error in=w1364) -> (error out=w1360:errorcluster, "Value"=w1356:string)  [unwired: 1 in, 1 out]
        n508 = call "Log File Root Properties.vi"("error in"=w1360, "Author"=w1357, "Description"=w1358, "Title"=w1356) -> ("error out"=w1359:errorcluster, "Author"=w1353:string, "Description"=w1354:string, "Title"=w1355:string)  [unwired: 4 in]
        n509 = property on="Title" class="Str"(error in=w1359, "Value"=w1355) -> (error out=w1361:errorcluster)  [unwired: 1 in, 1 out]
        n510 = property on="Description" class="Str"(error in=w1361, "Value"=w1354) -> (error out=w1362:errorcluster)  [unwired: 1 in, 1 out]
        n511 = property on="Author" class="Str"(error in=w1362, "Value"=w1353) -> (error out=w1363:errorcluster)  [unwired: 1 in, 1 out]
      }
      frame "CSV Delimiter" {
        n512 = property on="delimiter" class="Str"(error in=w1369) -> (error out=w1373:errorcluster, "Value"=w1371:string)  [unwired: 1 in, 1 out]
        n513 = call "Delimiter.vi"("error in"=w1373, "Delimiter"=w1371) -> ("error out"=w1372:errorcluster, "Delimiter"=w1370:string)  [unwired: 8 in]
        n514 = property on="delimiter" class="Str"(error in=w1372, "Value"=w1370) -> (error out=w1368:errorcluster)  [unwired: 1 in, 1 out]
      }
      frame "DB Type" {
        n515 = property on="DB Type" class="DigNum (strict)"(error in=w1375) -> (error out=w1377:errorcluster, "Value"=w1376:u16)  [unwired: 1 in, 1 out]
        n516 = call "Database Type.vi"("error in"=w1377, "DB Type"=w1376) -> ("error out"=w1383:errorcluster, "DB Type"=w1382:u16)  [unwired: 8 in]
        n517 = property on="DB Type" class="DigNum (strict)"(error in=w1383, "Value"=w1382) -> (error out=w1380:errorcluster)  [unwired: 1 in, 1 out]
        n518 = call-poly "General Enqueue Function - Data Logger.vi"("QRef in"=w1379, "Array of Messages"=T13[] [{"state"=enum."initialize 6", "data"=variant}, {"state"=enum."initialize 7", "data"=variant}, {"state"=enum."Idle", "data"=variant}], "Error in"=w1380) -> ("Error out"=w1381:errorcluster)  [unwired: 11 in, 1 out]
      }
      frame "Hidden Processes" {
        n519 = property on="Server Name" class="Str"(error in=w1393) -> (error out=w1392:errorcluster, "Value"=w1391:string)  [unwired: 1 in, 1 out]
        n520 = property on="Invisible Libraries" class="Arr (strict)"(error in=w1392) -> (error out=w1397:errorcluster, "Value"=w1395:string[])  [unwired: 1 in, 1 out]
        n521 = call "Invisible Processes.vi"("error in"=w1397, "Server Name"=w1391, "Current Hiden Processes"=w1395) -> ("error out"=w1396:errorcluster, "Invis Libraries"=w1394:string[])  [unwired: 7 in]
        n522 = property on="Invisible Libraries" class="Arr (strict)"(error in=w1396, "Val(Sgnl)"=w1394) -> (error out=w1387:errorcluster)  [unwired: 1 in, 1 out]
        n523 = property on="Deployed Libraries" class="LstBox (strict)"(error in=w1387, "Value"=i32[] [0] ("Deployed Libraries")) -> (error out=w1386:errorcluster)  [unwired: 1 in, 1 out]
        n524 = call-poly "General Enqueue Function - Data Logger.vi"("QRef in"=w1389, "Array of Messages"=T13[] [{"state"=enum."initialize 4", "data"=variant}, {"state"=enum."initialize 5", "data"=variant}, {"state"=enum."initialize 6", "data"=variant}, {"state"=enum."initialize 7", "data"=variant}, {"state"=enum."Idle", "data"=variant}], "Error in"=w1386) -> ("Error out"=w1390:errorcluster)  [unwired: 11 in, 1 out]
      }
      frame "Save to config file" {
        n525 = Variant To Data(error in=w1409, type=enum16{"App", "User"}."App", Variant=w1408) -> (data=w1406:enum16{"App", "User"}, error out=w1405:errorcluster)
        n526 = case shown="\"App\"" w1406 {
          selector: w1406 -> [w1420 w1431]
          tunnel: [w1423 FALSE] -> w1404
          tunnel: [w1422 w1430] -> w1400
          tunnel: [w1421 w1428] -> w1403
          tunnel: [w1420 w1431] -> _
          tunnel: w1405 -> [w1418 w1428]
          tunnel: w1401 -> [w1417 w1427]
          tunnel: [w1417 w1427] -> w1399
          frame "User", Default {
            n527 = call "File Dialog3"("prompt"="Select a new or existing file" ("default name"), "button label"="Save", "default name"="Config File", "error in"=w1418, "pattern (all files)"="*.ini") -> ("selected path"=w1422:path, "cancelled"=w1423:bool, "error out"=w1421:errorcluster)  [unwired: 7 in, 1 out]
          }
          frame "App" {
            n528 = call "Data logger Default Paths.vi"("Path Type"=enum16{"Config File", "Image File"}."Config File") -> ("Path"=w1430:path)  [unwired: 4 in]
          }
        }
        n529 = case shown="False" w1404 {
          tunnel: w1403 -> [w1412 w1416]
          tunnel: [w1411 w1415] -> w1402
          tunnel: w1400 -> [w1414 _]
          tunnel: w1399 -> [w1413 _]
          frame False {
            n530 = call "Data Logging Save Config.vi"("error in (no error)"=w1412, "Cluster"=w1413, "Path"=w1414) -> ("error out"=w1411:errorcluster)  [unwired: 8 in]
          }
          frame True {
            n531 = call <vilib>:"Clear Errors.vi"("error in (no error)"=w1416) -> ("error out"=w1415:errorcluster)  [unwired: 5 in, 1 out]
          }
        }
      }
      frame "Open from config file" {
        n532 = Variant To Data(error in=w1443, type=enum16{"App", "User"}."App", Variant=w1442) -> (data=w1440:enum16{"App", "User"}, error out=w1439:errorcluster)
        n533 = case shown="\"App\"" w1440 {
          selector: w1440 -> [w1454 w1465]
          tunnel: [w1457 FALSE] -> w1438
          tunnel: [w1456 w1464] -> w1434
          tunnel: [w1455 w1462] -> w1437
          tunnel: [w1454 w1465] -> _
          tunnel: w1439 -> [w1452 w1462]
          tunnel: w1435 -> [w1451 w1461]
          tunnel: [w1451 w1461] -> w1433
          frame "User", Default {
            n534 = call "File Dialog4"("prompt"="Select a config file" ("default name"), "button label"="Open", "default name"="Config File", "error in"=w1452, "pattern (all files)"="*.ini") -> ("selected path"=w1456:path, "cancelled"=w1457:bool, "error out"=w1455:errorcluster)  [unwired: 7 in, 1 out]
          }
          frame "App" {
            n535 = call "Data logger Default Paths.vi"("Path Type"=enum16{"Config File", "Image File"}."Config File") -> ("Path"=w1464:path)  [unwired: 4 in]
          }
        }
        n536 = case shown="False" w1438 {
          tunnel: w1437 -> [w1447 w1450]
          tunnel: [w1446 w1449] -> w1436
          tunnel: w1434 -> [w1448 _]
          tunnel: w1433 -> [w1445 _]
          frame False {
            n537 = call "Data Logger Open Config.vi"("error in"=w1447, "Cluster"=w1445, "Path"=w1448) -> ("error out"=w1446:errorcluster)  [unwired: 8 in]
          }
          frame True {
            n538 = call <vilib>:"Clear Errors.vi"("error in (no error)"=w1450) -> ("error out"=w1449:errorcluster)  [unwired: 5 in, 1 out]
          }
        }
      }
      frame "Logged File Viewer" {
        n539 = call "Under Construction.vi"("error in (no error)"=w1468) -> ("error out"=w1467:errorcluster)  [unwired: 10 in]
      }
      frame "Exit" {
        n540 = Not(x=w1472) -> (.not. x?=w1471:bool)
      }
    }
    n541 = call "Data Logger Error Handling.vi"("error in"=w1305, "Enum"=enum16{"Main", "Event", "Config"}."Config") -> ("error out"=w1304:errorcluster)  [unwired: 7 in]
    n542 = Or(x=w1304, y=w1311) -> (x .or. y?=w1312:bool)
  }
  n543 = Merge Errors(w96, w95, w61) -> (w67:errorcluster)
  n544 = call "Release Queues.vi"("error in (no error)"=w67, "Q3"=w64, "Q2 Cluster"=w65, "Q1"=w66) -> ("error out"=w27:errorcluster)  [unwired: 7 in]
  n545 = call <userlib>:"Dispose Notification Icon.vi"("NotifyIcon in"=w25, "error in (no error)"=w27) -> ("error out"=w28:errorcluster)  [unwired: 13 out]
  n546 = Unregister For Events(event registration refnum=w24, error in=w28) -> (error out=w26:errorcluster)
  n547 = call "App Closing.vi"("erro"=w26, "milliseconds to wait"=u32 1000) -> ()  [unwired: 9 in, 1 out]
